vi "Main.vi"() -> ()   [LabVIEW 2024, in "FlexiFlowInterfaceCH2.lvlib"]
doc: "This template is based from the Queued Message Handler design pattern and the Queued Message Handler Project Template that ships with LabVIEW 2014.\n\nThe main difference is that the Queue is private to this module and communication between modules is done via Broadcast and Request events.\n\nRequest events are wrapped via public API methods and are handled in the Event handler loop in this VI.\nAny module can register for Broadcast events sent by this module.\n\nThe Event Handling Loop generates messages based on user interface actions.\n\nThe Message Handling Loop processes messages generated by the Event Handling Loop, or by other messages. The messages are string values, so new messages can be added easily to the Message Cases case structure in the Message Handling Loop. Each message cluster can also provide an optional value for Message Data, which is a variant that can be converted to whatever message-specific data is required.\n_____\nBased on Delacor QMH Project Template 3.1.0.34."
uses:
  FlexiFlowInterfaceCH2.lvlib
  <vilib>/Delacor/Delacor QMH/Libraries/Module Admin_class/Delacor_lib_QMH_Module Admin.lvclass
  <vilib>/MGI/Panel Manager/Panel/Panel/Panel.lvclass
  Module Data--cluster.ctl
  Modbus TCP Connection Settings--cluster.ctl
  Modbus Flexi-Flow State--cluster.ctl
  <vilib>/Plasmionique/MB Master/MB_Master_TCP/MB_Master_TCP.lvclass
  C:/Program Files/National Instruments/LabVIEW 2025/vi.lib/Plasmionique/MB Master/MB_Master/MB_Master.lvclass
  Device Type--enum.ctl
  Modbus Flexi-Flow Controls--cluster.ctl
  Modbus Flexi-Flow API/Control Mode--enum.ctl
  Modbus Flexi-Flow API/Control Function Values--enum.ctl
  Modbus Flexi-Flow Measure State--cluster.ctl
  <vilib>/Utility/miscctls.llb/LVPointTypeDef.ctl
  Initialise Modbus Connections Argument--cluster.ctl
  <vilib>/Delacor/Delacor QMH/Libraries/Message Queue_class/Delacor_lib_QMH_Message Queue.lvclass/Delacor_lib_QMH_Message Queue.ctl
  Stop Argument--cluster.ctl
  <vilib>/Delacor/Delacor QMH/Libraries/Module Admin_class/Delacor_lib_QMH_Module Admin.lvclass/Delacor_lib_QMH_Module Admin.ctl
  Read Fmeasure Argument--cluster.ctl
  FlexiFlowDevice--enum.ctl
  Set Modbus Configuration Argument--cluster.ctl
  Wink Devices Argument--cluster.ctl
  Read All FlexiFlow Device States Argument--cluster.ctl
  Wink Device Argument--cluster.ctl
  Set Control Function Argument--cluster.ctl
  Set Flow Setpoint Argument--cluster.ctl
  Set Backpressure Setpoint Argument--cluster.ctl
  Set Forward Pressure SP Argument--cluster.ctl
  Set Flow Capacity Unit Argument--cluster.ctl
  Modbus Flexi-Flow API/Capacity Units (Standard Volume Flow).ctl
  Set Setpoint Slope Argument--cluster.ctl
  Set Counter Settings Argument--cluster.ctl
  Counter Settings--cluster.ctl
  Modbus Flexi-Flow API/Counter Setpoint Mode--enum.ctl
  Modbus Flexi-Flow API/Counter Modes--enum.ctl
  Reset All Device Counters Argument--cluster.ctl
  Read Device User Tag Argument--cluster.ctl
  Set Device User Tag Argument--cluster.ctl
  Read Counter Unit Argument--cluster.ctl
  Set Control Mode Argument--cluster.ctl
  Get Device Configuration Argument--cluster.ctl
  Modbus Flexi-Flow API/PDU Address Float 32-bit Params--ring.ctl
  <vilib>/Delacor/Delacor QMH/Libraries/Message Queue_class/Delacor_lib_QMH_Enqueue Message (Single).vi
  <vilib>/Delacor/Delacor QMH/Libraries/Module Admin_class/Delacor_lib_QMH_Get External Launch.vi
  <vilib>/Utility/error.llb/Error Cluster From Error Code.vi
  <vilib>/ErrorRing/Error Ring.xnode
  <vilib>/Delacor/Delacor QMH/Libraries/Message Queue_class/Delacor_lib_QMH_Message Queue.lvclass
  <vilib>/MGI/Panel Manager/Panel/Panel Helper/Panel Helper.lvclass
  Modbus Flexi-Flow API/Bronkhorst Flexi-Flow ModbusTCP API.lvlib
panel:
  out "Counter Unit":string
  out "Read Capacity Unit":string
  out "Counters":sgl[](array[numeric])
  in  "Flexi-Flow Conn":T1[](array[typedef])=[{"Label"="hydrogen_inlet", "Slave ID (255)"=255, "IP Address"="192.168.100.10", "Port (502)"=502, "Timeout (10000)"=2000}, {"Label"="nitrogen_inlet", "Slave ID (255)"=255, "IP Address"="192.168.100.20", "Port (502)"=502, "Timeout (10000)"=2000}, {"Label"="cathode_outlet", "Slave ID (255)"=255, "IP Address"="192.168.100.30", "Port (502)"=502, "Timeout (10000)"=2000}, {"Label"="anode_outlet", "Slave ID (255)"=255, "IP Address"="192.168.100.40", "Port (502)"=502, "Timeout (10000)"=2000}]
  out "Data Cluster":T2 {"Flexi-Flow Devices"."Control State"."Control Mode" items=["Bus/RS232"=0, "FLOW-BUS slave"=2, "Valve close"=3, "Controller idle"=4, "Setpoint 100%"=7, "Valve fully open"=8, "Calibration mode"=9, "Setpoint 0%"=12, "RS232"=18, "Valve steering"=20, "Valve safe state"=22]}
  in  "Panel":refnum<class "Panel.lvclass">
  in  "Simulate MHL Error":bool
  in  "Simulate EHL Error":bool
  out "error out":errorcluster
  in  "Module Admin":refnum<class "Delacor_lib_QMH_Module Admin.lvclass">
  out "Status":string
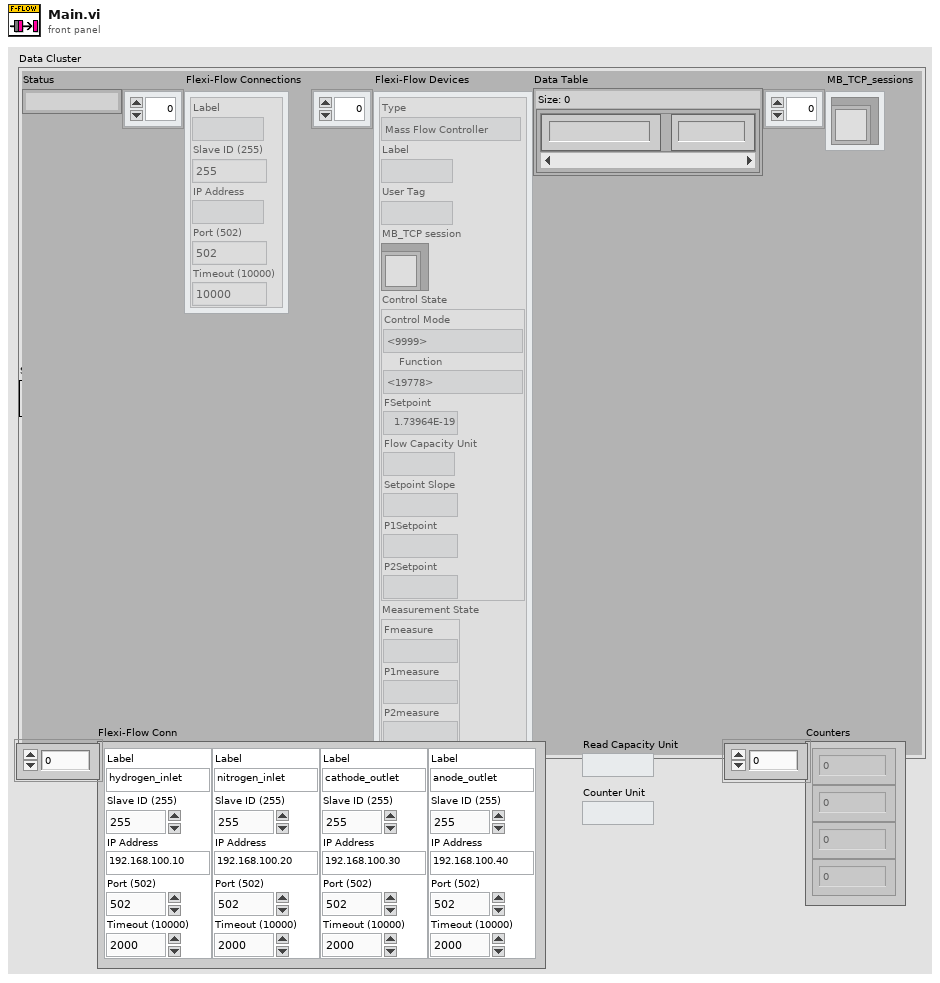
[diagram p1: front panel]
types:
  T1 = typedef "FlexiFlowInterfaceCH2.lvlib/Modbus TCP Connection Settings--cluster.ctl" = cluster{"Label":string, "Slave ID (255)":u8, "IP Address":string, "Port (502)":u16, "Timeout (10000)":i32}
  T2 = typedef "FlexiFlowInterfaceCH2.lvlib/Module Data--cluster.ctl" = cluster{"Status":string, "Flexi-Flow Connections":T1[], "Flexi-Flow Devices":T3[], "Data Table":map{string, dbl}, "MB_TCP_sessions":refnum<class "MB_Master_TCP.lvclass">[]}
  T3 = typedef "FlexiFlowInterfaceCH2.lvlib/Modbus Flexi-Flow State--cluster.ctl" = cluster{"Type":T4, "Label":string, "User Tag":string, "MB_TCP session":refnum<class "MB_Master_TCP.lvclass">, "Control State":T5, "Measurement State":T8}
  T4 = typedef "FlexiFlowInterfaceCH2.lvlib/Device Type--enum.ctl" = enum16{"Mass Flow Controller", "Mass Flow Meter"}
  T5 = typedef "FlexiFlowInterfaceCH2.lvlib/Modbus Flexi-Flow Controls--cluster.ctl" = cluster{"Control Mode":T6, "Function":T7, "FSetpoint":sgl, "Flow Capacity Unit":string, "Setpoint Slope":u16, "P1Setpoint":sgl, "P2Setpoint":sgl}
  T6 = typedef "Bronkhorst Flexi-Flow ModbusTCP API.lvlib/Control Mode--enum.ctl" = u16
  T7 = typedef "Bronkhorst Flexi-Flow ModbusTCP API.lvlib/Control Function Values--enum.ctl" = enum16{"Flow", "Upstream pressure", "Downstream pressure", "Flow with upstream pressure limit", "Flow with downstream pressure limit", "Upstream pressure with flow limit", "Downstream pressure with flow limit"}
  T8 = typedef "FlexiFlowInterfaceCH2.lvlib/Modbus Flexi-Flow Measure State--cluster.ctl" = cluster{"Fmeasure":dbl, "P1measure":sgl, "P2measure":sgl}
  T9 = typedef "LVPointTypeDef.ctl" = cluster{"Horizontal":i16, "Vertical":i16}
  T10 = typedef "FlexiFlowInterfaceCH2.lvlib/Request Events--cluster.ctl" = cluster{"Stop Module":refnum<user-event>, "Show Panel":refnum<user-event>, "Hide Panel":refnum<user-event>, "Get Module Execution Status":refnum<user-event>, "Show Diagram":refnum<user-event>, "Change Panel":refnum<user-event>, "Private":cluster{"Start Modbus Polling Helper Loop":refnum<user-event>, "Sleep Modbus Polling Helper Loop":refnum<user-event>, "Wake Connection Helper Loop":refnum<user-event>, "Sleep Connection Helper Loop":refnum<user-event>}, "Initialise Modbus Connections":refnum<user-event>, "Read Fmeasure":refnum<user-event>, "Set Modbus Configuration":refnum<user-event>, "Wink Devices":refnum<user-event>, "Read All FlexiFlow Device States":refnum<user-event>, "Wink Device":refnum<user-event>, "Set Control Function":refnum<user-event>, "Set Flow Setpoint":refnum<user-event>, "Set Backpressure Setpoint":refnum<user-event>, "Set Forward Pressure SP":refnum<user-event>, "Set Capacity Unit":refnum<user-event>, "Set Flow Capacity Unit":refnum<user-event>, "Set Setpoint Slope":refnum<user-event>, "Set Counter Settings":refnum<user-event>, "Reset All Device Counters":refnum<user-event>, "Read Device User Tag":refnum<user-event>, "Set Device User Tag":refnum<user-event>, "Read Counter Unit":refnum<user-event>, "Set Control Mode":refnum<user-event>, "Get Device Configuration":refnum<user-event>}
  T11 = typedef "Panel.lvlib/Panel Helper.lvclass/Panel Events.ctl" = cluster{"My Panel":refnum<user-event>, "Top Level Initialized":refnum<user-event>}
  T12 = typedef "FlexiFlowInterfaceCH2.lvlib/Initialise Modbus Connections Argument--cluster.ctl" = cluster{"Boolean":bool}
  T13 = typedef "FlexiFlowInterfaceCH2.lvlib/Stop Argument--cluster.ctl" = cluster{"Origin":string, "Exit via Stop Module Req?":bool, "Wait for Module to stop?":bool}
  T14 = typedef "FlexiFlowInterfaceCH2.lvlib/Read Fmeasure Argument--cluster.ctl" = cluster{"Device":T15}
  T15 = typedef "FlexiFlowInterfaceCH2.lvlib/FlexiFlowDevice--enum.ctl" = enum16{"Hydrogen Inlet", "Nitrogen Inlet", "Cathode Outlet", "Anode Outlet"}
  T16 = typedef "FlexiFlowInterfaceCH2.lvlib/Set Modbus Configuration Argument--cluster.ctl" = cluster{"Device":T15, "Modbus TCP Connection":T1}
  T17 = typedef "FlexiFlowInterfaceCH2.lvlib/Wink Devices Argument--cluster.ctl" = cluster{"Boolean":bool}
  T18 = typedef "FlexiFlowInterfaceCH2.lvlib/Read All FlexiFlow Device States Argument--cluster.ctl" = cluster{"Boolean":bool}
  T19 = typedef "FlexiFlowInterfaceCH2.lvlib/Wink Device Argument--cluster.ctl" = cluster{"Device":T15}
  T20 = typedef "FlexiFlowInterfaceCH2.lvlib/Set Control Function Argument--cluster.ctl" = cluster{"Device":T15, "Function":T7}
  T21 = typedef "FlexiFlowInterfaceCH2.lvlib/Set Flow Setpoint Argument--cluster.ctl" = cluster{"Device":T15, "Setpoint Value":dbl}
  T22 = typedef "FlexiFlowInterfaceCH2.lvlib/Set Backpressure Setpoint Argument--cluster.ctl" = cluster{"Device":T15, "Backpressure SP":dbl}
  T23 = typedef "FlexiFlowInterfaceCH2.lvlib/Set Forward Pressure SP Argument--cluster.ctl" = cluster{"Device":T15, "Pressure SP":dbl}
  T24 = typedef "FlexiFlowInterfaceCH2.lvlib/Set Flow Capacity Unit Argument--cluster.ctl" = cluster{"Device":T15, "Standard Volume Flow":T25}
  T25 = typedef "Bronkhorst Flexi-Flow ModbusTCP API.lvlib/Capacity Units (Standard Volume Flow).ctl" = u16
  T26 = typedef "FlexiFlowInterfaceCH2.lvlib/Set Setpoint Slope Argument--cluster.ctl" = cluster{"Setpoint Slope":u16, "Device":T15}
  T27 = typedef "FlexiFlowInterfaceCH2.lvlib/Set Counter Settings Argument--cluster.ctl" = cluster{"Device":T15, "Counter Settings":T28}
  T28 = typedef "FlexiFlowInterfaceCH2.lvlib/Counter Settings--cluster.ctl" = cluster{"Counter Setpoint Mode":T29, "Counter Limit":sgl, "Unit":string, "Counter Mode":T30, "Counter New Setpoint":u16}
  T29 = typedef "Bronkhorst Flexi-Flow ModbusTCP API.lvlib/Counter Setpoint Mode--enum.ctl" = enum16{"No setpoint change (default)", "Change setpoint to Counter new setpoint"}
  T30 = typedef "Bronkhorst Flexi-Flow ModbusTCP API.lvlib/Counter Modes--enum.ctl" = enum16{"Counter off (default)", "Counting up continuously", "Counting up until limit reached"}
  T31 = typedef "FlexiFlowInterfaceCH2.lvlib/Reset All Device Counters Argument--cluster.ctl" = cluster{"Boolean":bool}
  T32 = typedef "FlexiFlowInterfaceCH2.lvlib/Read Device User Tag Argument--cluster.ctl" = cluster{"Device":T15}
  T33 = typedef "FlexiFlowInterfaceCH2.lvlib/Set Device User Tag Argument--cluster.ctl" = cluster{"Device":T15, "User Tag":string}
  T34 = typedef "FlexiFlowInterfaceCH2.lvlib/Read Counter Unit Argument--cluster.ctl" = cluster{"Device":T15}
  T35 = typedef "FlexiFlowInterfaceCH2.lvlib/Set Control Mode Argument--cluster.ctl" = cluster{"Device":T15, "Control Mode":T6}
  T36 = typedef "FlexiFlowInterfaceCH2.lvlib/Get Device Configuration Argument--cluster.ctl" = cluster{"Device":T15}
  T37 = enum32{"invalid lock state", "Not Locked", "Locked (No Password)", "Password-protected"}
  T38 = enum16{"No reset", "Reset counter", "Reset alarm", "Reset counter (all)", "Reset and disable counter", "Reset firmware program (soft reset)", "Reset Alarm infor error bit", "Reset Alarm info warning bit"}
  T39 = typedef "Bronkhorst Flexi-Flow ModbusTCP API.lvlib/PDU Address Float 32-bit Params--ring.ctl" = u16
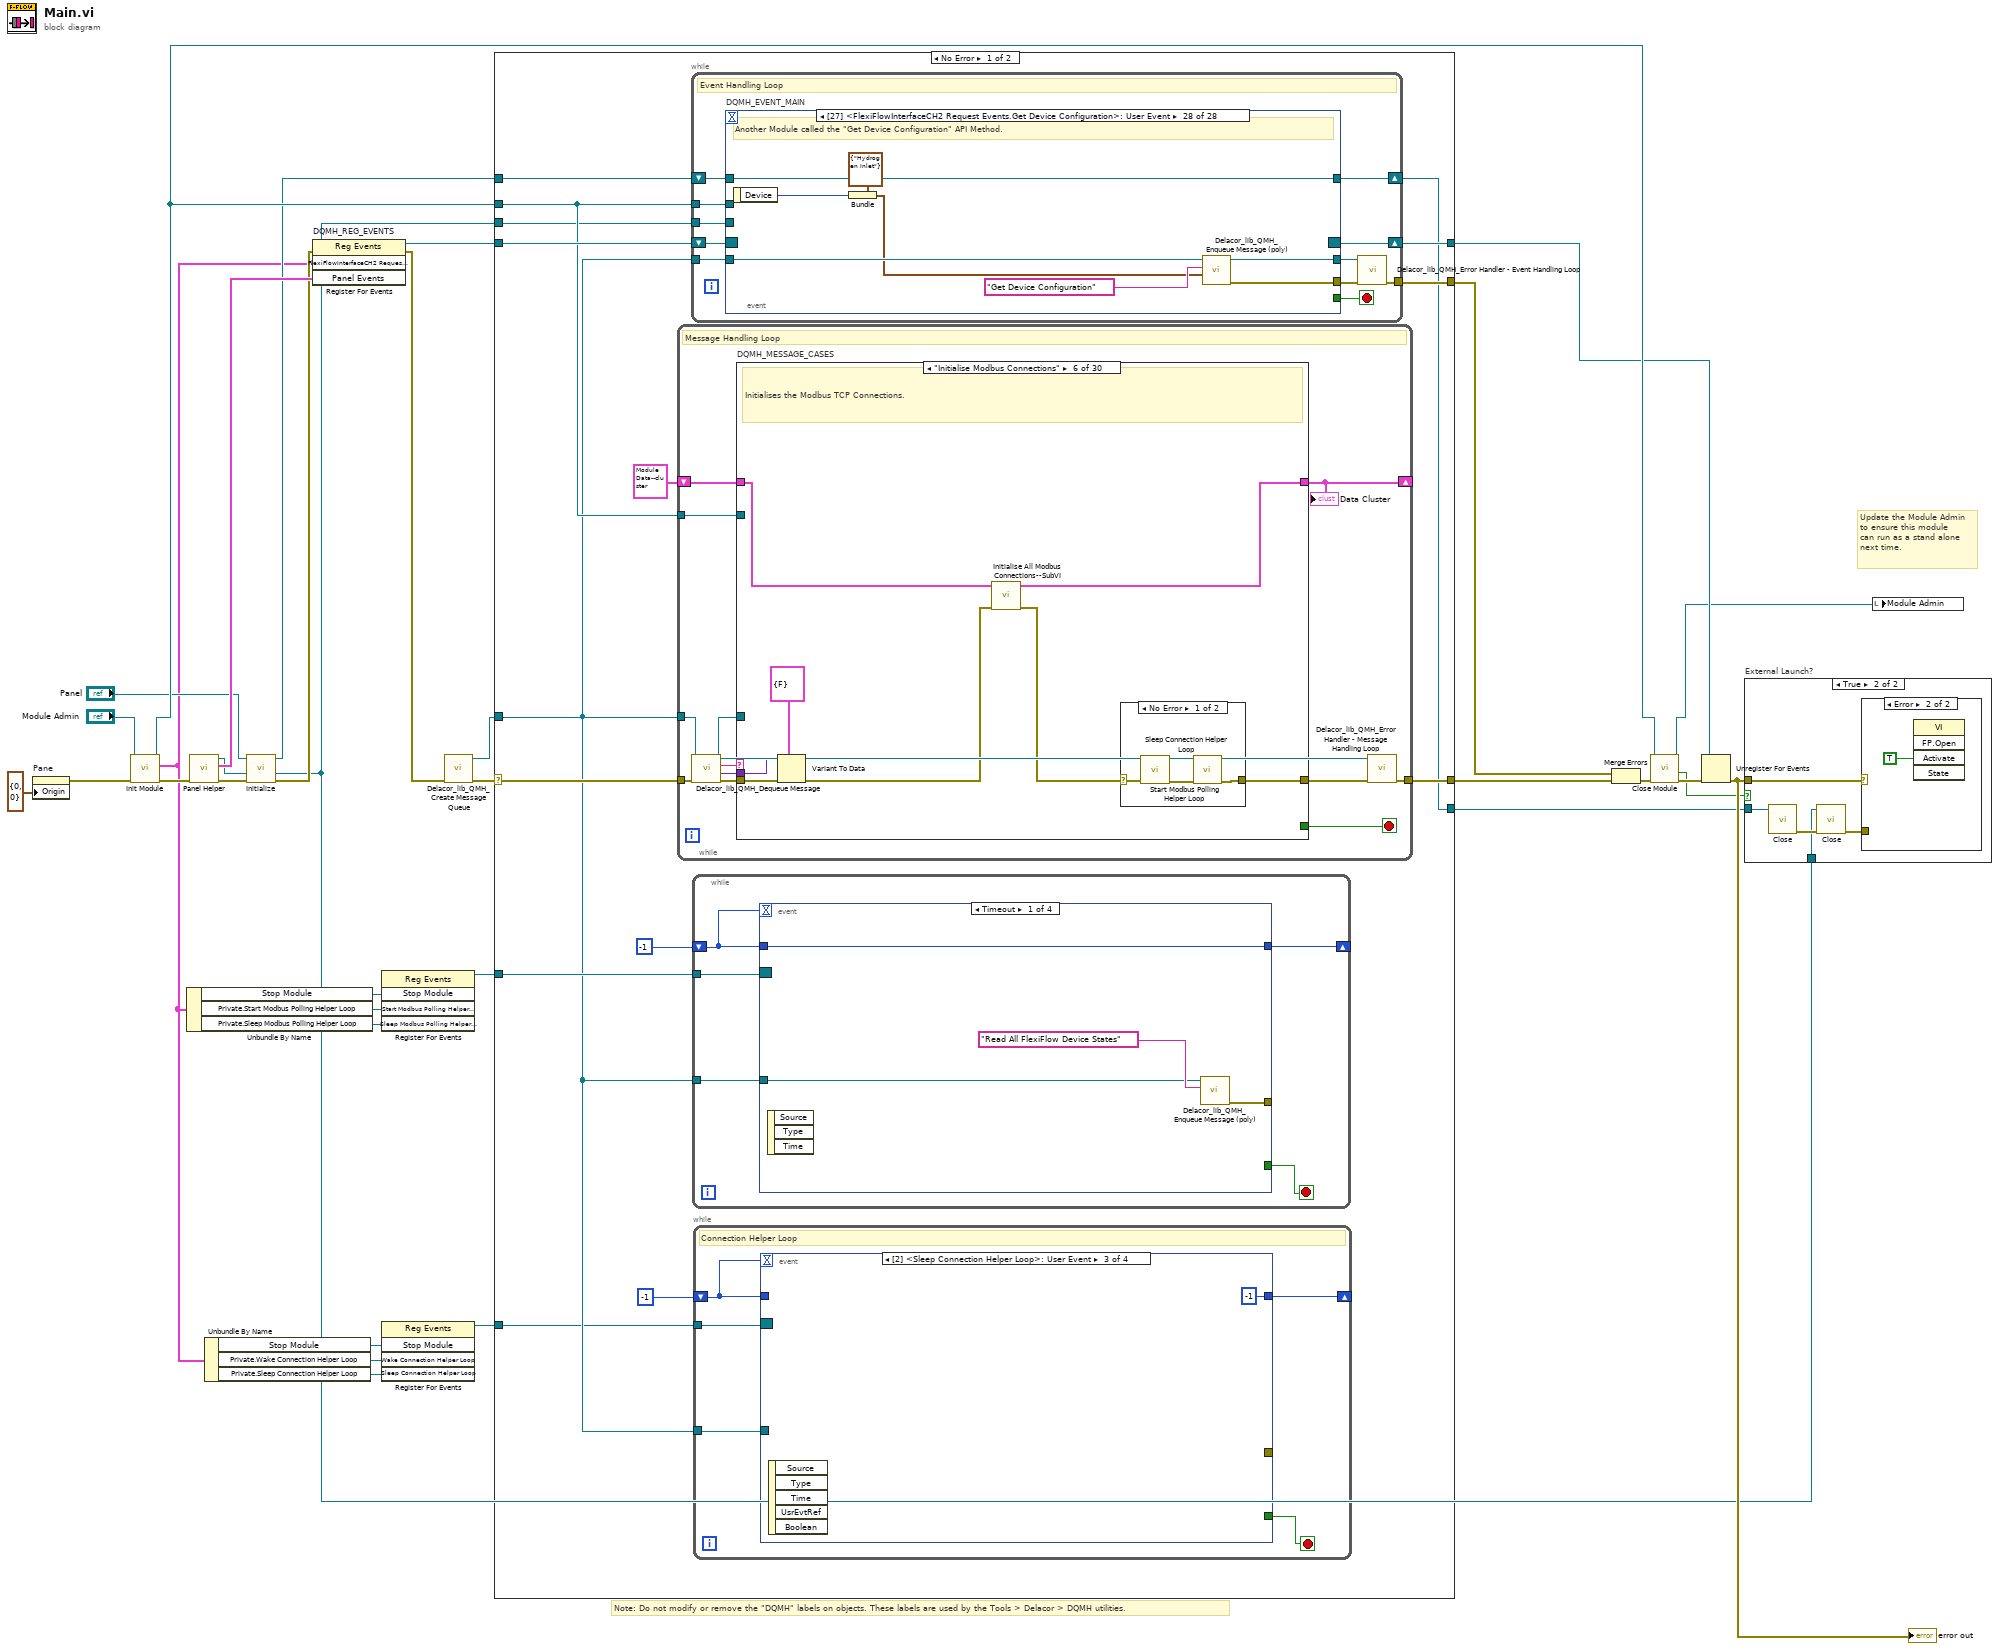
[diagram p0: block diagram]
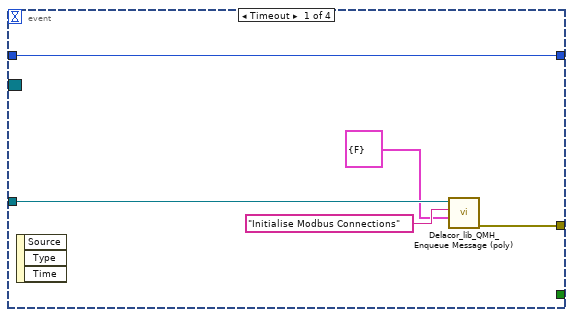
[diagram p4: hidden frame]
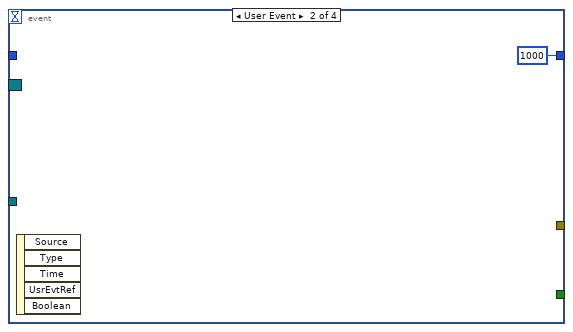
[diagram p5: hidden frame]
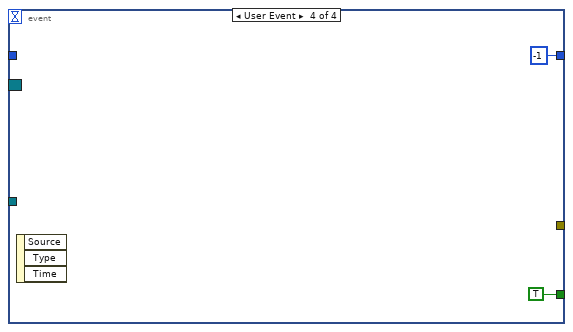
[diagram p6: hidden frame]
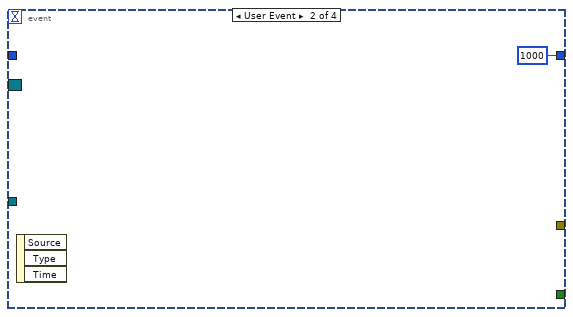
[diagram p7: hidden frame]
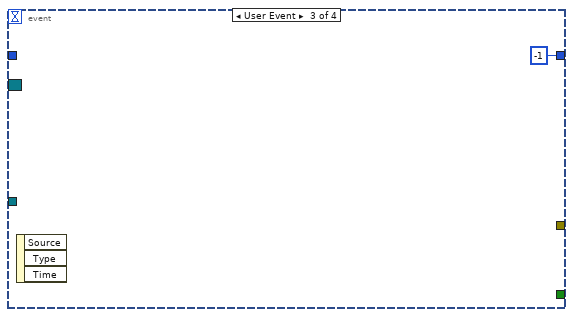
[diagram p8: hidden frame]
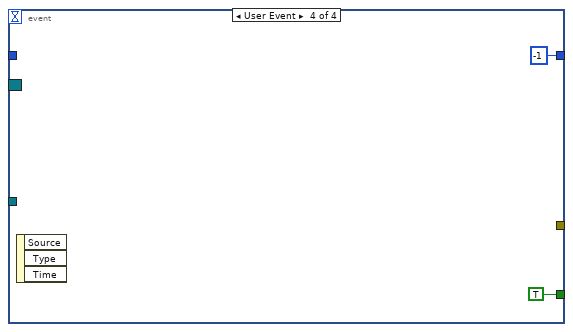
[diagram p9: hidden frame]
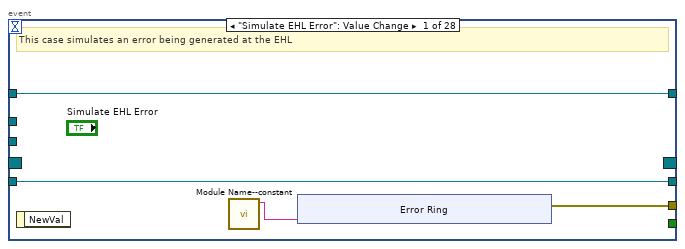
[diagram p10: hidden frame]
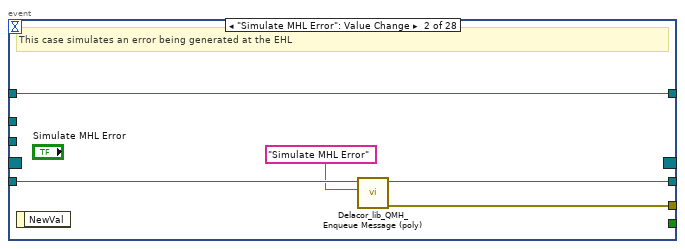
[diagram p11: hidden frame]
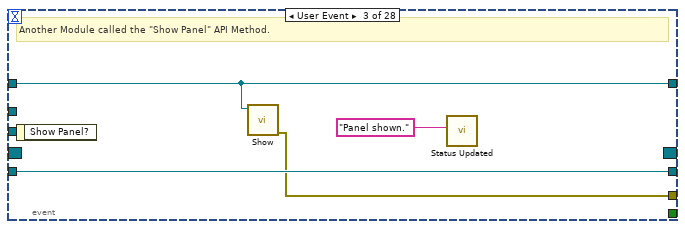
[diagram p12: hidden frame]
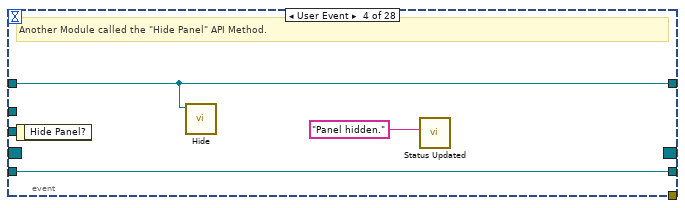
[diagram p13: hidden frame]
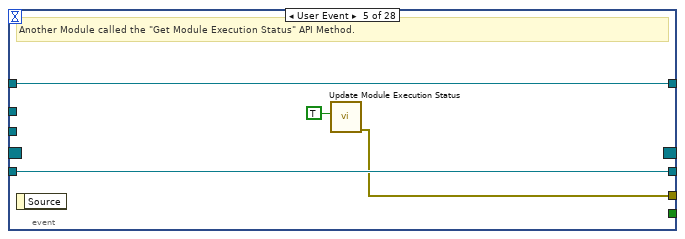
[diagram p14: hidden frame]
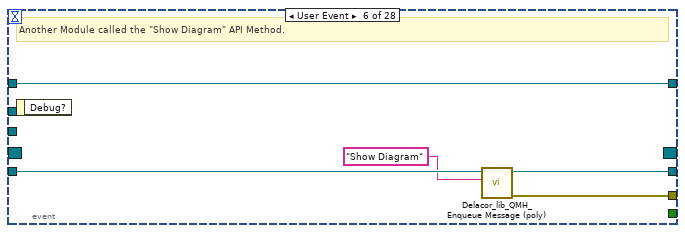
[diagram p15: hidden frame]
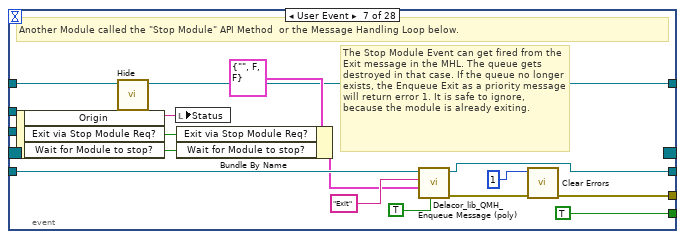
[diagram p16: hidden frame]
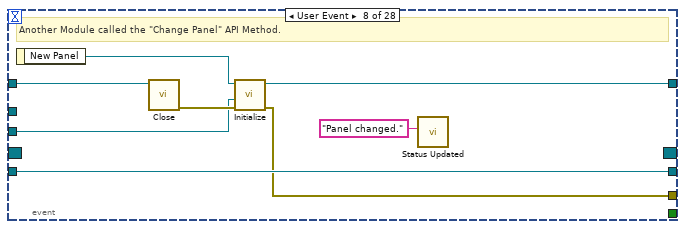
[diagram p17: hidden frame]
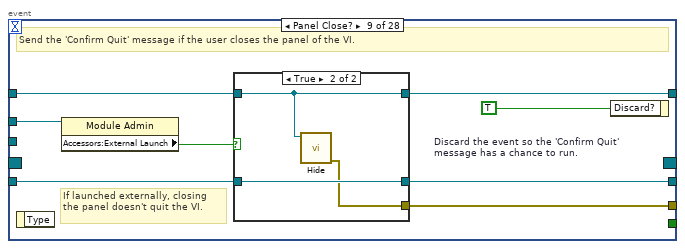
[diagram p18: hidden frame]
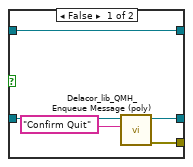
[diagram p19: hidden frame]
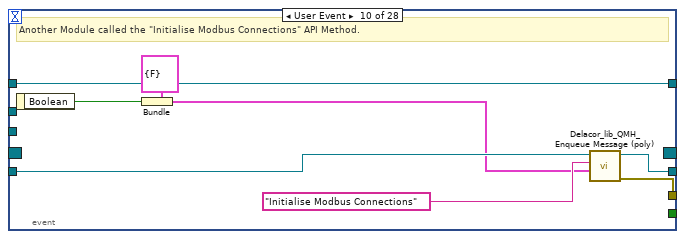
[diagram p20: hidden frame]
diagram:
  # "Note: Do not modify or remove the \"DQMH\" labels on objects. These labels are used by the Tools > Delacor > DQMH utilities."
  # "Update the Module Admin to ensure this module can run as a stand alone next time."
  n1 = property on="Pane" class="Pane"("Origin"=T9 {"Horizontal"=0, "Vertical"=0}) -> (error out=w10:errorcluster)  [unwired: 2 in, 1 out]
  n2 = call "Init Module.vi"("error in (no error)"=w10, "Singleton Module Admin in"="Module Admin") -> ("error out"=w20:errorcluster, "FlexiFlowInterfaceCH2 Request Events"=w5:T10, "Singleton Module Admin out"=w34:refnum<class "Delacor_lib_QMH_Module Admin.lvclass">)  [unwired: 7 in]
  n3 = Unbundle By Name(w5) -> ("Stop Module"=w8:refnum<user-event>, "Private.Start Modbus Polling Helper Loop"=w7:refnum<user-event>, "Private.Sleep Modbus Polling Helper Loop"=w6:refnum<user-event>)
  n4 = call <vilib>:"Panel Helper.vi"("Error In"=w20) -> ("Error Out"=w17:errorcluster, "Panel Events"=w19:T11, "Panel Helper out"=w16:refnum<class "Panel Helper.lvclass">)  [unwired: 8 in]
  n5 = Unbundle By Name(w5) -> ("Stop Module"=w4:refnum<user-event>, "Private.Wake Connection Helper Loop"=w3:refnum<user-event>, "Private.Sleep Connection Helper Loop"=w1:refnum<user-event>)
  n6 = call <vilib>:"Initialize.vi"("error in (no error)"=w17, "My Helper in"=w16, "Panel In"="Panel") -> ("error out"=w14:errorcluster, "My Helper out"=w13:refnum<class "Panel Helper.lvclass">, "Panel Out"=w12:refnum<class "Panel.lvclass">)  [unwired: 6 in]
  n7 = register-events "DQMH_REG_EVENTS"(error in=w14, w5, w19) -> (reference out=w31:refnum<event-registration>, error out=w18:errorcluster)  [unwired: 1 in]
  n8 = register-events(w8, w7, w6) -> (reference out=w9:refnum<event-registration>)  [unwired: 2 in, 1 out]
  n9 = register-events(w4, w3, w1) -> (reference out=w2:refnum<event-registration>)  [unwired: 2 in, 1 out]
  n10 = call <vilib>:"Delacor_lib_QMH_Create Message Queue.vi"("error in"=w18) -> ("error out"=w22:errorcluster, "Message Queue"=w30:refnum<class "Delacor_lib_QMH_Message Queue.lvclass">)  [unwired: 9 in]
  n11 = case shown="No Error" w22 {
    selector: w22 -> [w44 w707]
    tunnel: [w49 w707] -> w33
    tunnel: [w48 w712] -> w32
    tunnel: w31 -> [w46 w712]
    tunnel: w30 -> [w36 _]
    tunnel: [w45 _] -> w26
    tunnel: w34 -> [w43 w708]
    tunnel: w12 -> [w41 w704]
    tunnel: w13 -> [w42 _]
    tunnel: [w40 w704] -> w21
    tunnel: w9 -> [w38 _]
    tunnel: w2 -> [w35 _]
    frame No Error {
      n12 = while {
        tunnel: w36 -> [w324]
        shift-right: [w320] -> _
        shift-left: T2 {"Status"="", "Flexi-Flow Connections"=[], "Flexi-Flow Devices"=[], "Data Table"={}, "MB_TCP_sessions"=[]} ("Data Cluster") -> [w330]
        tunnel: w44 -> [w328]
        tunnel: [w322] -> w49
        tunnel: w43 -> [w321]
        stop <- w329 stop-if-true
        # "Message Handling Loop"
        n13 = call-dynamic "Delacor_lib_QMH_Dequeue Message.vi"("error in"=w328, "Message Queue in"=w324) -> ("error out"=w327:errorcluster, "Message Data"=w325:variant, "Message"=w326:string, "Message Queue out"=w323:refnum<class "Delacor_lib_QMH_Message Queue.lvclass">)  [unwired: 6 in]
        n14 = case "DQMH_MESSAGE_CASES" shown="\"Initialise Modbus Connections\"" w326 {
          selector: w326 -> [_ _ _ _ _ _ _ _ _ _ _ _ _ _ _ _ _ _ _ _ _ _ _ _ _ _ _ _ _ w694]
          tunnel: w323 -> [_ _ _ _ _ _ _ _ _ _ _ _ _ _ _ _ _ _ _ _ _ _ _ _ _ _ w654 w669 w687 _]
          tunnel: w327 -> [w341 w351 w355 w372 w378 w386 w399 w412 w428 w441 w457 w476 w495 w506 w516 w524 w543 w552 w574 w588 w602 w617 w631 w634 w637 w642 w659 w672 w689 _]
          tunnel: [w342 w352 w354 w371 w377 w380 w396 w407 w423 w437 w450 w467 w485 w502 w510 w520 w536 w544 w566 w578 w590 w604 w618 w633 w636 w641 w651 w671 w684 w695] -> w331
          tunnel: w330 -> [w338 w345 w353 w370 w373 w382 w394 w405 w420 w436 w453 w469 w484 w498 w512 w523 w539 w549 w568 w582 w596 w609 w625 w632 w635 w638 w650 w666 w675 w692]
          tunnel: [_ _ _ _ _ _ _ _ _ _ _ _ _ _ _ _ _ _ _ _ _ _ _ _ _ _ _ _ w686 _] -> w329
          tunnel: w325 -> [_ w350 _ _ w376 w385 w398 w411 w427 w440 w456 w475 w494 w505 w515 w526 w542 w551 w573 w587 w601 w616 w630 _ _ _ w658 _ w683 _]
          tunnel: w321 -> [w339 _ _ _ _ _ _ _ _ _ _ _ _ _ _ _ _ _ _ _ _ _ _ _ _ _ w653 _ w678 _]
          tunnel: [w336 w345 w353 w370 w373 w381 w393 w404 w418 w430 w449 w463 w483 w500 w508 w522 w538 w548 w563 w581 w595 w608 w624 w632 w635 w638 w650 w666 w675 w692] -> w320
          frame "Initialize" {
            w337 = "Initial Message" ("Initial Message")
            # "Initialize - Any operation that needs to be done before the module can receive messages. Synchronize Caller Events.vi will inform Start Module.vi that the module has launched and is ready to receive messages. Module Did Init.vi will broadcast that the module initialized."
            n15 = Array Size(array="Flexi-Flow Conn") -> (size(s)=w333:i32)
            n16 = local write "Status"(w337) -> ()
            n17 = Initialize Array(T3 {"Type"=enum."Mass Flow Controller", "Label"="", "User Tag"="", "MB_TCP session"=refnum, "Control State"={"Control Mode"=0, "Function"=enum."Flow", "FSetpoint"=0.0, "Flow Capacity Unit"="", "Setpoint Slope"=0, "P1Setpoint"=0.0, "P2Setpoint"=0.0}, "Measurement State"={"Fmeasure"=0.0, "P1measure"=0.0, "P2measure"=0.0}} ("Flexi-Flow"), w333) -> (w332:T3[])
            n18 = call "Synchronize Caller Events.vi"("error in (no error)"=w341, "Singleton Module Admin in"=w339) -> ("error out"=w340:errorcluster)  [unwired: 8 in, 1 out]
            n19 = Bundle By Name(cluster=w338, "Status"=w337, "Flexi-Flow Connections"="Flexi-Flow Conn", "Flexi-Flow Devices"=w332) -> (w336:T2)
            n20 = call "Module Name--constant.vi"() -> ("Module Name"=w343:string)  [unwired: 11 in]
            n21 = call "Module Did Init.vi"("error in (no error)"=w340, "Initialized?"=TRUE, "Origin"=w343) -> ("error out"=w342:errorcluster)  [unwired: 8 in]
          }
          frame "Update Display" {
            # "Broadcast updated status to any VI registered to listen to this module's broadcast events."
            # "Convert the message data to a string to display in the Status indicator."
            # "#CodeRecommended - If you wish to decouple the Message Handling Loop from your user interface, consider creating User Events (like the \"Stop\" event in this VI) to message the Event Handling Loop whenever the user interface needs updating."
            # "Update Display - Update user interface here."
            n22 = Variant To Data(error in=w351, type="" ("Empty String Constant"), Variant=w350) -> (data=w348:string, error out=w347:errorcluster)
            "Status" <- w348
            n23 = call "Status Updated.vi"("error in (no error)"=w347, "Status"=w348) -> ("error out"=w346:errorcluster)  [unwired: 9 in]
            n24 = Merge Errors(w346) -> (w352:errorcluster)
          }
          frame "Show Diagram" {
            # "Show Diagram - Show the block diagram of this VI. Used as a debugging tool. There is a button in the module tester that fires the Show Diagram request, which runs this message. Note that the diagram will not be displayed if it is password-protected and the password is not in the cache."
            n25 = disable-structure shown="RUN_TIME_ENGINE==False" {
              disable-tunnel: [w363 w369] -> w354
              disable-tunnel: w355 -> [w362 w369]
              frame condition #0 (active) {
                # "functionality not available in exe"
                n26 = invoke class="VI" method="Lock State.Get"(error in=w362) -> (error out=w361:errorcluster, "Get Lock State"=w360:T37, "pwd in cache"=w357:bool)  [unwired: 3 in, 1 out]
                n27 = Equal?(x=T37."Password-protected", y=w360) -> (x = y?=w358:bool)
                n28 = Compound Arithmetic op=AND(w358, invert w357) -> (w356:bool)
                n29 = case shown="False" w356 {
                  tunnel: [w366 w368] -> w363
                  tunnel: w361 -> [w364 w368]
                  frame False {
                    n30 = property class="VI"(error in=w364, "BDWin.Open"=TRUE ("Block Diagram Window:Open")) -> (error out=w366:errorcluster)  [unwired: 1 in, 1 out]
                    n31 = call "Status Updated.vi"("Status"="Block Diagram shown." ("format string")) -> ()  [unwired: 10 in, 1 out]
                  }
                  frame True {
                    # "Password-protected VI, and the password is not in the cache. Do not show the diagram."
                  }
                }
              }
              frame condition #1 {
              }
            }
          }
          frame "--- Module Specific ---" {
            # "Separator -- The following cases handle messages specific to this Module."
            n32 = Merge Errors(w372) -> (w371:errorcluster)
          }
          frame "Set Modbus Configuration" {
            # "Sets the modbus configuration."
            n33 = Variant To Data(error in=w378, type=T16 {"Device"=enum."Hydrogen Inlet", "Modbus TCP Connection"={"Label"="", "Slave ID (255)"=255, "IP Address"="", "Port (502)"=502, "Timeout (10000)"=10000}} ("Set Modbus Configuration Argument"), Variant=w376) -> (data=w374:T16, error out=w377:errorcluster)
            n34 = Unbundle By Name(w374) -> ()  [unwired: 2 out]
          }
          frame "Initialise Modbus Connections" {
            # "Initialises the Modbus TCP Connections."
            n35 = Variant To Data(error in=w386, type=T12 {"Boolean"=FALSE} ("Initialise Modbus Connections Argument"), Variant=w385) -> (error out=w383:errorcluster)  [unwired: 1 out]
            n36 = call "Initialise All Modbus Connections--SubVI.vi"("error in (no error)"=w383, "Data Cluster in"=w382) -> ("error out"=w379:errorcluster, "Data Cluster out"=w381:T2)  [unwired: 8 in]
            n37 = case shown="No Error" w379 {
              selector: w379 -> [w388 w392]
              tunnel: [w389 w390] -> w380
              frame No Error {
                n38 = call "Sleep Connection Helper Loop.vi"("error in"=w388) -> ("error out"=w387:errorcluster)  [unwired: 10 in]
                n39 = call "Start Modbus Polling Helper Loop.vi"("error in"=w387) -> ("error out"=w389:errorcluster)  [unwired: 10 in]
              }
              frame Error {
                n40 = call "Sleep Modbus Polling Helper Loop.vi"("error in"=w392) -> ("error out"=w391:errorcluster)  [unwired: 10 in]
                n41 = call "Wake Connection Helper Loop.vi"("error in"=w391) -> ("error out"=w390:errorcluster)  [unwired: 10 in]
              }
            }
          }
          frame "Wink Devices" {
            # "Wink the flexi-flow devices."
            n42 = Variant To Data(error in=w399, type=T17 {"Boolean"=FALSE} ("Wink Devices Argument"), Variant=w398) -> (error out=w395:errorcluster)  [unwired: 1 out]
            n43 = call "Wink Devices--SubVI.vi"("error in (no error)"=w395, "Data Cluster in"=w394) -> ("error out"=w396:errorcluster, "Data Cluster out"=w393:T2)  [unwired: 8 in]
          }
          frame "Wink Device" {
            # "Winks the specified FlexiFlow device."
            n44 = Variant To Data(error in=w412, type=T19 {"Device"=enum."Hydrogen Inlet"} ("Wink Device Argument"), Variant=w411) -> (data=w409:T19, error out=w408:errorcluster)
            n45 = Unbundle By Name(w409) -> ("Device"=w400:T15)
            n46 = call "Get Device Modbus TCP Session.vi"("Device"=w400, "Data Cluster In"=w405) -> ("Device State"=w401:T3, "MB_TCP session"=w402:refnum<class "MB_Master_TCP.lvclass">, "Data Cluster Out"=w406:T2)  [unwired: 7 in]
            n47 = call "Wink.vi"("error in"=w408, "MB_TCP session in"=w402) -> ("error out"=w407:errorcluster, "MB session out"=w403:refnum<class "MB_Master_TCP.lvclass">)  [unwired: 8 in]
            n48 = call "Update Device.vi"("Device"=w400, "Device State"=w401, "MB_TCP session"=w403, "Data Cluster"=w406) -> ("Data Cluster Out"=w404:T2)  [unwired: 7 in]
          }
          frame "Set Control Function" {
            # "Sets the control function."
            n49 = Variant To Data(error in=w428, type=T20 {"Device"=enum."Hydrogen Inlet", "Function"=enum."Flow"} ("Set Control Function Argument"), Variant=w427) -> (data=w425:T20, error out=w424:errorcluster)
            n50 = Unbundle By Name(w425) -> ("Device"=w414:T15, "Function"=w422:T7)
            n51 = call "Get Device Modbus TCP Session.vi"("Device"=w414, "Data Cluster In"=w420) -> ("Device State"=w416:T3, "MB_TCP session"=w415:refnum<class "MB_Master_TCP.lvclass">, "Data Cluster Out"=w421:T2)  [unwired: 7 in]
            n52 = call "Write Control Function.vi"("error in"=w424, "Function"=w422, "MB_TCP session in"=w415) -> ("error out"=w423:errorcluster, "Value"=w419:u16, "MB session out"=w413:refnum<class "MB_Master_TCP.lvclass">)  [unwired: 6 in]
            n53 = Bundle By Name(cluster=w416, "Control State.Function"=w419) -> (w417:T3)
            n54 = call "Update Device.vi"("Device"=w414, "Device State"=w417, "MB_TCP session"=w413, "Data Cluster"=w421) -> ("Data Cluster Out"=w418:T2)  [unwired: 7 in]
          }
          frame "Set Counter Settings" {
            # "Set the counter settings."
            n55 = Variant To Data(error in=w441, type=T27 {"Device"=enum."Hydrogen Inlet", "Counter Settings"={"Counter Setpoint Mode"=enum."No setpoint change (default)", "Counter Limit"=0.0, "Unit"="ls", "Counter Mode"=enum."Counter off (default)", "Counter New Setpoint"=0}} ("Set Counter Settings Argument"), Variant=w440) -> (data=w432:T27, error out=w438:errorcluster)
            n56 = Unbundle By Name(w432) -> ("Device"=w431:T15)
            n57 = call "Get Device Modbus TCP Session.vi"("Device"=w431, "Data Cluster In"=w436) -> ("Device State"=w434:T3, "MB_TCP session"=w429:refnum<class "MB_Master_TCP.lvclass">, "Data Cluster Out"=w435:T2)  [unwired: 7 in]
            n58 = call "Set Counter Settings--SubVI.vi"("error in (no error)"=w438, "Set Counter Settings Argument"=w432, "MB_Master_TCP in"=w429) -> ("error out"=w437:errorcluster, "MB_Master_TCP out"=w433:refnum<class "MB_Master_TCP.lvclass">)  [unwired: 7 in]
            n59 = call "Update Device.vi"("Device"=w431, "Device State"=w434, "MB_TCP session"=w433, "Data Cluster"=w435) -> ("Data Cluster Out"=w430:T2)  [unwired: 7 in]
          }
          frame "Set Flow Setpoint" {
            # "Sets the control value setpoint."
            n60 = Variant To Data(error in=w457, type=T21 {"Device"=enum."Hydrogen Inlet", "Setpoint Value"=0.0} ("Set Control Value SP Argument"), Variant=w456) -> (data=w454:T21, error out=w451:errorcluster)
            n61 = Unbundle By Name(w454) -> ("Device"=w444:T15, "Setpoint Value"=w452:dbl)
            n62 = call "Get Device Modbus TCP Session.vi"("Device"=w444, "Data Cluster In"=w453) -> ("Device State"=w446:T3, "MB_TCP session"=w445:refnum<class "MB_Master_TCP.lvclass">, "Data Cluster Out"=w448:T2)  [unwired: 7 in]
            n63 = call "Write Fsetpoint (Channel F).vi"("error in"=w451, "Value"=w452, "MB_TCP session in"=w445) -> ("error out"=w450:errorcluster, "Value"=w447:sgl, "MB session out"=w442:refnum<class "MB_Master_TCP.lvclass">)  [unwired: 6 in]
            n64 = Bundle By Name(cluster=w446, "Control State.FSetpoint"=w447) -> (w443:T3)
            n65 = call "Update Device.vi"("Device"=w444, "Device State"=w443, "MB_TCP session"=w442, "Data Cluster"=w448) -> ("Data Cluster Out"=w449:T2)  [unwired: 7 in]
          }
          frame "Set Backpressure Setpoint" {
            w465 = T39 41496 items=["FSetpoint (Channel F)"=41240, "Fmeasure (Channel F)"=41216, "FSetpoint (Channel P1)"=41496, "Fmeasure (Channel P1)"=41472, "FSetpoint (Channel P2)"=41752, "Fmeasure (Channel P2)"=41728, "Capacity 0%"=41392, "Counter limit (Float)"=59416, "Inlet Pressure"=61801, "Outlet Pressure"=61809, "PID-Kp"=62120, "PID-Ti"=62128, "PID-Td"=62136, "Dynamic display factor"=62728, "Static display factor"=62736, "Exponential smoothing"=62752] ("PDU Address 32-bit Float")
            # "Sets the backpressure setpoint (P1 - upstream) of the pressure regulator."
            n66 = Variant To Data(error in=w476, type=T22 {"Device"=enum."Cathode Outlet", "Backpressure SP"=0.0} ("Set Backpressure Setpoint Argument"), Variant=w475) -> (data=w473:T22, error out=w472:errorcluster)
            n67 = Unbundle By Name(w473) -> ("Device"=w462:T15, "Backpressure SP"=w471:dbl)
            n68 = call "Get Device Modbus TCP Session.vi"("Device"=w462, "Data Cluster In"=w469) -> ("Device State"=w461:T3, "MB_TCP session"=w460:refnum<class "MB_Master_TCP.lvclass">, "Data Cluster Out"=w470:T2)  [unwired: 7 in]
            n69 = call "Write Float Register.vi"("PDU Address 32-bit Float"=w465, "error in"=w472, "Value"=w471, "MB_TCP session in"=w460) -> ("error out"=w468:errorcluster, "MB session out"=w466:refnum<class "MB_Master_TCP.lvclass">)  [unwired: 6 in]
            n70 = call "Read Float Register.vi"("PDU Address 32-bit Float"=w465, "error in"=w468, "MB_TCP session in"=w466) -> ("error out"=w467:errorcluster, "Value"=w464:sgl, "MB session out"=w459:refnum<class "MB_Master_TCP.lvclass">)  [unwired: 6 in]
            n71 = Bundle By Name(cluster=w461, "Control State.P1Setpoint"=w464) -> (w458:T3)
            n72 = call "Update Device.vi"("Device"=w462, "Device State"=w458, "MB_TCP session"=w459, "Data Cluster"=w470) -> ("Data Cluster Out"=w463:T2)  [unwired: 7 in]
          }
          frame "Set Forward Pressure SP" {
            w482 = T39 41752 items=["FSetpoint (Channel F)"=41240, "Fmeasure (Channel F)"=41216, "FSetpoint (Channel P1)"=41496, "Fmeasure (Channel P1)"=41472, "FSetpoint (Channel P2)"=41752, "Fmeasure (Channel P2)"=41728, "Capacity 0%"=41392, "Counter limit (Float)"=59416, "Inlet Pressure"=61801, "Outlet Pressure"=61809, "PID-Kp"=62120, "PID-Ti"=62128, "PID-Td"=62136, "Dynamic display factor"=62728, "Static display factor"=62736, "Exponential smoothing"=62752] ("PDU Address 32-bit Float")
            # "Sets the forward pressure setpoint."
            n73 = Variant To Data(error in=w495, type=T23 {"Device"=enum."Hydrogen Inlet", "Pressure SP"=0.0} ("Set Forward Pressure SP Argument"), Variant=w494) -> (data=w492:T23, error out=w486:errorcluster)
            n74 = Unbundle By Name(w492) -> ("Device"=w480:T15, "Pressure SP"=w487:dbl)
            n75 = call "Get Device Modbus TCP Session.vi"("Device"=w480, "Data Cluster In"=w484) -> ("Device State"=w479:T3, "MB_TCP session"=w481:refnum<class "MB_Master_TCP.lvclass">, "Data Cluster Out"=w491:T2)  [unwired: 7 in]
            n76 = call "Write Float Register.vi"("PDU Address 32-bit Float"=w482, "error in"=w486, "Value"=w487, "MB_TCP session in"=w481) -> ("error out"=w490:errorcluster, "MB session out"=w489:refnum<class "MB_Master_TCP.lvclass">)  [unwired: 6 in]
            n77 = call "Read Float Register.vi"("PDU Address 32-bit Float"=w482, "error in"=w490, "MB_TCP session in"=w489) -> ("error out"=w485:errorcluster, "Value"=w488:sgl, "MB session out"=w477:refnum<class "MB_Master_TCP.lvclass">)  [unwired: 6 in]
            n78 = Bundle By Name(cluster=w479, "Control State.P2Setpoint"=w488) -> (w478:T3)
            n79 = call "Update Device.vi"("Device"=w480, "Device State"=w478, "MB_TCP session"=w477, "Data Cluster"=w491) -> ("Data Cluster Out"=w483:T2)  [unwired: 7 in]
          }
          frame "Set Flow Capacity Unit" {
            # "Sets the flow capacity unit."
            n80 = Variant To Data(error in=w506, type=T24 {"Device"=enum."Hydrogen Inlet", "Standard Volume Flow"=0} ("Set Flow Capacity Unit Argument"), Variant=w505) -> (data=w503:T24, error out=w501:errorcluster)
            n81 = Unbundle By Name(w503) -> ("Device"=w497:T15, "Standard Volume Flow"=w496:T25)
            n82 = call "Set Flow Capacity Unit--SubVI.vi"("error in (no error)"=w501, "Standard Volume Flow"=w496, "Device"=w497, "Data Cluster"=w498) -> ("error out"=w502:errorcluster, "Value"=→"Read Capacity Unit":string, "Data Cluster Out"=w500:T2)  [unwired: 5 in]
          }
          frame "Set Setpoint Slope" {
            # "Sets the setpoint slope in seconds. 0 to 3000 seconds. 0 is default. 10 corresponds to a change from 0 to 100% over 10 seconds."
            n83 = Variant To Data(error in=w516, type=T26 {"Setpoint Slope"=0, "Device"=enum."Hydrogen Inlet"} ("Set Setpoint Slope Argument"), Variant=w515) -> (data=w513:T26, error out=w511:errorcluster)
            n84 = Unbundle By Name(w513) -> ("Device"=w509:T15, "Setpoint Slope"=w507:u16)
            n85 = call "Set Setpoint Slope--SubVI.vi"("error in (no error)"=w511, "Setpoint Slope"=w507, "Device"=w509, "Data Cluster"=w512) -> ("error out"=w510:errorcluster, "Data Cluster Out"=w508:T2)  [unwired: 6 in]
          }
          frame "Read All FlexiFlow Device States" {
            # "Reads all Flex-Flow device states."
            n86 = Variant To Data(error in=w524, type=T18 {"Boolean"=FALSE} ("Read All FlexiFlow Device States Argument"), Variant=w526) -> ()  [unwired: 2 out]
            n87 = call "Read All Devices States.vi"("error in (no error)"=w524, "Data Cluster"=w523) -> ("error out"=w517:errorcluster, "Array"=→"Counters":sgl[], "Data Table"=w519:map{string, dbl}, "Array Out"=w521:T3[])  [unwired: 6 in]
            n88 = case shown="Error .." w517 {
              selector: w517 -> [w527 w534]
              tunnel: w521 -> [w531 _]
              tunnel: [w529 w532] -> w520
              tunnel: w519 -> [w528 _]
              frame No Error {
                n89 = call "Broadcast Device States.vi"("error in"=w527, "Flexi-Flow Devices"=w531) -> ("error out"=w530:errorcluster)  [unwired: 9 in]
                n90 = call "Broadcast State (Data Map).vi"("error in"=w530, "Data Table"=w528) -> ("error out"=w529:errorcluster)  [unwired: 9 in]
              }
              frame Error {
                n91 = call "Wake Connection Helper Loop.vi"("error in"=w534) -> ("error out"=w533:errorcluster)  [unwired: 10 in]
                n92 = call "Sleep Modbus Polling Helper Loop.vi"("error in"=w533) -> ("error out"=w532:errorcluster)  [unwired: 10 in]
              }
            }
            n93 = Bundle By Name(cluster=w523, "Flexi-Flow Devices"=w521, "Data Table"=w519) -> (w522:T2)
          }
          frame "Read Measure" {
            n94 = Variant To Data(error in=w543, type=T14 {"Device"=enum."Hydrogen Inlet"} ("Read Device State Argument"), Variant=w542) -> (data=w540:T14, error out=w537:errorcluster)
            n95 = Unbundle By Name(w540) -> ("Device"=w535:T15)
            n96 = call "Read Measure--SubVI.vi"("error in (no error)"=w537, "Device"=w535, "Data Cluster"=w539) -> ("error out"=w536:errorcluster, "Data Cluster Out"=w538:T2)  [unwired: 7 in]
          }
          frame "Reset All Device Counters" {
            # "Resets all device counters."
            n97 = Variant To Data(error in=w552, type=T31 {"Boolean"=FALSE} ("Reset All Device Counters Argument"), Variant=w551) -> (error out=w545:errorcluster)  [unwired: 1 out]
            n98 = Unbundle By Name(w549) -> ("Flexi-Flow Devices"=w547:T3[])
            n99 = for {
              tunnel: w547 -> [w558] mode=indexing
              tunnel: [w556] -> w546 mode=indexing
              tunnel: w545 -> [w554]
              tunnel: [w553] -> w544
              n100 = Unbundle By Name(w558) -> ("MB_TCP session"=w559:refnum<class "MB_Master_TCP.lvclass">)
              n101 = call "Write Reset.vi"("error in"=w554, "Reset Arguments"=T38."Reset counter (all)", "MB_TCP session in"=w559) -> ("error out"=w553:errorcluster, "MB session out"=w557:refnum<class "MB_Master_TCP.lvclass">)  [unwired: 7 in]
              n102 = Bundle By Name(cluster=w558, "MB_TCP session"=w557) -> (w556:T3)
            }
            n103 = Bundle By Name(cluster=w549, "Flexi-Flow Devices"=w546) -> (w548:T2)
          }
          frame "Read Device User Tag" {
            # "Reads the user tag of the device."
            n104 = Variant To Data(error in=w574, type=T32 {"Device"=enum."Hydrogen Inlet"} ("Read Device User Tag Argument"), Variant=w573) -> (data=w571:T32, error out=w567:errorcluster)
            n105 = Unbundle By Name(w571) -> ("Device"=w569:T15)
            n106 = call "Get Device Modbus TCP Session.vi"("Device"=w569, "Data Cluster In"=w568) -> ("Device State"=w562:T3, "MB_TCP session"=w564:refnum<class "MB_Master_TCP.lvclass">, "Data Cluster Out"=w570:T2)  [unwired: 7 in]
            n107 = call "Read User Tag.vi"("error in"=w567, "MB_TCP session in"=w564) -> ("error out"=w566:errorcluster, "Value"=w560:string, "MB session out"=w565:refnum<class "MB_Master_TCP.lvclass">)  [unwired: 7 in]
            n108 = Bundle By Name(cluster=w562, "User Tag"=w560) -> (w561:T3)
            n109 = call "Update Device.vi"("Device"=w569, "Device State"=w561, "MB_TCP session"=w565, "Data Cluster"=w570) -> ("Data Cluster Out"=w563:T2)  [unwired: 7 in]
          }
          frame "Set Device User Tag" {
            # "Sets the device user tag."
            n110 = Variant To Data(error in=w588, type=T33 {"Device"=enum."Hydrogen Inlet", "User Tag"=""} ("Set Device User Tag Argument"), Variant=w587) -> (data=w585:T33, error out=w579:errorcluster)
            n111 = Unbundle By Name(w585) -> ("Device"=w580:T15, "User Tag"=w575:string)
            n112 = call "Get Device Modbus TCP Session.vi"("Device"=w580, "Data Cluster In"=w582) -> ("Device State"=w583:T3, "MB_TCP session"=w577:refnum<class "MB_Master_TCP.lvclass">, "Data Cluster Out"=w584:T2)  [unwired: 7 in]
            n113 = call "Write User Tag.vi"("error in"=w579, "Label"=w575, "MB_TCP session in"=w577) -> ("error out"=w578:errorcluster, "MB session out"=w576:refnum<class "MB_Master_TCP.lvclass">)  [unwired: 7 in]
            n114 = call "Update Device.vi"("Device"=w580, "Device State"=w583, "MB_TCP session"=w576, "Data Cluster"=w584) -> ("Data Cluster Out"=w581:T2)  [unwired: 7 in]
          }
          frame "Read Counter Unit" {
            # "#CodeNeeded\n1. Configure this Message Case for handling the \"Read Counter Unit\" message.\n2. Delete or edit this label when done."
            # "Reads the counter unit."
            n115 = Variant To Data(error in=w602, type=T34 {"Device"=enum."Hydrogen Inlet"} ("Read Counter Unit Argument"), Variant=w601) -> (data=w599:T34, error out=w591:errorcluster)
            n116 = Unbundle By Name(w599) -> ("Device"=w594:T15)
            n117 = call "Get Device Modbus TCP Session.vi"("Device"=w594, "Data Cluster In"=w596) -> ("Device State"=w597:T3, "MB_TCP session"=w593:refnum<class "MB_Master_TCP.lvclass">, "Data Cluster Out"=w598:T2)  [unwired: 7 in]
            n118 = call "Read Counter Unit.vi"("error in"=w591, "MB_TCP session in"=w593) -> ("error out"=w590:errorcluster, "Value"=→"Counter Unit":string, "MB session out"=w592:refnum<class "MB_Master_TCP.lvclass">)  [unwired: 7 in]
            n119 = call "Update Device.vi"("Device"=w594, "Device State"=w597, "MB_TCP session"=w592, "Data Cluster"=w598) -> ("Data Cluster Out"=w595:T2)  [unwired: 7 in]
          }
          frame "Set Control Mode" {
            # "Sets the flexi-flow control mode."
            n120 = Variant To Data(error in=w617, type=T35 {"Device"=enum."Hydrogen Inlet", "Control Mode"=0} ("Set Control Mode Argument"), Variant=w616) -> (data=w614:T35, error out=w605:errorcluster)
            n121 = Unbundle By Name(w614) -> ("Device"=w610:T15, "Control Mode"=w603:T6)
            n122 = call "Get Device Modbus TCP Session.vi"("Device"=w610, "Data Cluster In"=w609) -> ("Device State"=w612:T3, "MB_TCP session"=w607:refnum<class "MB_Master_TCP.lvclass">, "Data Cluster Out"=w613:T2)  [unwired: 7 in]
            n123 = call "Write Control Mode.vi"("error in"=w605, "Control Mode"=w603, "MB_TCP session in"=w607) -> ("error out"=w604:errorcluster, "MB session out"=w606:refnum<class "MB_Master_TCP.lvclass">)  [unwired: 7 in]
            n124 = Bundle By Name(cluster=w612, "Control State.Control Mode"=w603) -> (w611:T3)
            n125 = call "Update Device.vi"("Device"=w610, "Device State"=w611, "MB_TCP session"=w606, "Data Cluster"=w613) -> ("Data Cluster Out"=w608:T2)  [unwired: 7 in]
          }
          frame "Get Device Configuration" {
            # "Gets the device configuration."
            n126 = Variant To Data(error in=w631, type=T36 {"Device"=enum."Hydrogen Inlet"} ("Get Device Configuration Argument"), Variant=w630) -> (data=w626:T36, error out=w619:errorcluster)
            n127 = Unbundle By Name(w626) -> ("Device"=w627:T15)
            n128 = call "Get Device Modbus TCP Session.vi"("Device"=w627, "Data Cluster In"=w625) -> ("Device State"=w621:T3, "MB_TCP session"=w623:refnum<class "MB_Master_TCP.lvclass">, "Data Cluster Out"=w628:T2)  [unwired: 7 in]
            n129 = call "Get Device Configuration--SubVI.vi"("error in (no error)"=w619, "Device State in"=w621, "MB_Master_TCP in"=w623) -> ("error out"=w618:errorcluster, "Device State out"=w620:T3, "MB_Master_TCP out"=w622:refnum<class "MB_Master_TCP.lvclass">)  [unwired: 6 in]
            n130 = call "Update Device.vi"("Device"=w627, "Device State"=w620, "MB_TCP session"=w622, "Data Cluster"=w628) -> ("Data Cluster Out"=w624:T2)  [unwired: 7 in]
          }
          frame "---Copy This Frame---" {
            # "Duplicate this frame when creating new messages.  Change this comment in the duplicated frame to describe this message."
            n131 = Merge Errors(w634) -> (w633:errorcluster)
          }
          frame "--- Exit and Error Handling---" {
            # "Separator - The following cases handle errors and exit messages."
            n132 = Merge Errors(w637) -> (w636:errorcluster)
          }
          frame "Simulate MHL Error" {
            # "Simulate an error occurring at the MHL"
            n133 = call "Module Name--constant.vi"() -> ("Module Name"=w640:string)  [unwired: 11 in]
            n134 = xnode "Error Ring"("parameter 0"=w640) -> ("error out"=w639:errorcluster)
            n135 = Merge Errors(w642, w639) -> (w641:errorcluster)
          }
          frame "Error" {
            # "#CodeRecommended - If you ever change the name of this \"Error\" message, you'll need to update the name in the Check Loop Error.vi as well."
            # "#CodeRecommended - If the module is running in standalone mode (External Launch = FALSE), this code will pop up an error dialog and call the 'Exit' message if an error occurs. Add more fine-grained error handling here."
            # "Error - Check the error message data and respond accordingly. This message is sent by the \"Error Handler\" VIs at the end of each loop in this application."
            n136 = property class="Module Admin"(reference=w653) -> ("Accessors:External Launch"=w652:bool)  [unwired: 1 in, 2 out]
            n137 = Variant To Data(error in=w659, type=errorcluster {"status"=FALSE, "code"=0, "source"=""} ("error constant"), Variant=w658) -> (data=w660:errorcluster, error out=w656:errorcluster)
            n138 = call "Error Reported.vi"("Error"=w660) -> ()  [unwired: 10 in, 1 out]
            n139 = case shown="False" w652 {
              tunnel: [w665 _] -> w655
              tunnel: w654 -> [w664 _]
              tunnel: w660 -> [w661 _]
              frame False {
                # "If the module is running standalone, then pop up an error dialog and call the \"Exit\" message."
                n140 = call <vilib>:"Simple Error Handler.vi"("error in (no error)"=w661) -> ()  [unwired: 4 in, 5 out]
                n141 = call-poly <vilib>:"Delacor_lib_QMH_Enqueue Message (poly).vi"("Priority Message? (F)"=TRUE, "Message"="Exit", "Message Queue in"=w664) -> ("error out"=w665:errorcluster)  [unwired: 7 in, 1 out]
              }
              frame True {
                # "If the module was launched externally, calling the Error Reported broadcast VI is the only action performed by the \"Error\" message. The module's caller can then process the error appropriately."
              }
            }
            n142 = Merge Errors(w656, w655) -> (w651:errorcluster)
            n143 = local write "error out"(w651) -> ()
          }
          frame "Confirm Quit" {
            # "#CodeNeeded - If you want to provide an \"Are you sure\" dialog (or some other notification) before the application exits, place that code here. This message is typically sent from a Panel Close? event."
            # "Confirm Quit - Message that can confirm whether or not the user wants to exit the application."
            n144 = call-poly <vilib>:"Delacor_lib_QMH_Enqueue Message (poly).vi"("Priority Message? (F)"=TRUE, "error in"=w672, "Message"="Exit", "Message Queue in"=w669) -> ("error out"=w670:errorcluster)  [unwired: 6 in, 1 out]
            n145 = Merge Errors(w670) -> (w671:errorcluster)
          }
          frame "Exit" {
            w681 = 91  # 91: not all Exit messages will have an argument
            w686 = TRUE  # Stop the VI
            # "Release the message queue reference"
            # "Exit - Exit the application."
            n146 = Variant To Data(error in=w689, type=T13 {"Origin"="", "Exit via Stop Module Req?"=FALSE, "Wait for Module to stop?"=FALSE} ("Stop Argument"), Variant=w683) -> (data=w679:T13, error out=w682:errorcluster)
            n147 = call <vilib>:"Clear Errors.vi"("error in (no error)"=w682, "specific error code to clear (0: all)"=w681) -> ("error out"=w688:errorcluster)  [unwired: 4 in, 1 out]
            n148 = Unbundle By Name(w675) -> ("MB_TCP_sessions"=w674:refnum<class "MB_Master_TCP.lvclass">[])
            n149 = call-dynamic "Delacor_lib_QMH_Release Message Queue.vi"("error in"=w688, "Message Queue"=w687) -> ("error out"=w685:errorcluster)  [unwired: 9 in]
            n150 = for {
              tunnel: [w691] -> w676
              tunnel: w674 -> [w690] mode=indexing
              n151 = call "Modbus TCP Close.vi"("MB session in"=w690) -> ("error out"=w691:errorcluster)  [unwired: 10 in]
            }
            n152 = call "Handle Exit.vi"("Stop Argument"=w679, "Admin in"=w678) -> ("error out"=w677:errorcluster)  [unwired: 8 in, 1 out]
            n153 = call "Sleep Modbus Polling Helper Loop.vi"() -> ("error out"=w673:errorcluster)  [unwired: 11 in]
            n154 = Merge Errors(w673, w677, w676, w685) -> (w684:errorcluster)
          }
          frame Default {
            # "'Default' case only runs if there is a message that isn't defined in any of the other cases.  Output a programming error."
            n155 = call "Module Name--constant.vi"() -> ("Module Name"=w693:string)  [unwired: 11 in]
            n156 = xnode "Error Ring"("parameter 0"=w694, "parameter 1"=w693) -> ("error out"=w695:errorcluster)
          }
        }
        "Data Cluster" <- w320
        n157 = call-dynamic "Delacor_lib_QMH_Error Handler - Message Handling Loop.vi"("error in"=w331, "Message Queue in"=w323) -> ("dup error in"=w322:errorcluster)  [unwired: 8 in, 1 out]
      }
      n158 = while {
        tunnel: w36 -> [w87]
        shift-right: [w85] -> w48
        shift-left: w46 -> [w86]
        tunnel: [w81] -> w45
        tunnel: w43 -> [w80]
        tunnel: w42 -> [w79]
        shift-right: [w77] -> w40
        shift-left: w41 -> [w78]
        stop <- w83 stop-if-true
        # "Event Handling Loop"
        n159 = event "DQMH_EVENT_MAIN" shown="[27] <FlexiFlowInterfaceCH2 Request Events.Get Device Configuration>: User Event" {
          selector: w86 -> [_ _ _ _ _ _ _ _ _ _ _ _ _ _ _ _ _ _ _ _ _ _ _ _ _ _ _ _]
          dyn-events: [_ _ _ _ _ _ _ _ _ _ _ _ _ _ _ _ _ _ _ _ _ _ _ _ _ _ _ _] -> w85
          timeout: _ -> [_ _ _ _ _ _ _ _ _ _ _ _ _ _ _ _ _ _ _ _ _ _ _ _ _ _ _ _]
          tunnel: [_ _ _ _ _ _ TRUE ("Discard?") _ _ _ _ _ _ _ _ _ _ _ _ _ _ _ _ _ _ _ _ _] -> w83
          tunnel: w87 -> [w91 w103 w107 w110 w114 w119 w131 w141 w148 w165 w173 w182 w190 w198 w206 w215 w224 w233 w242 w251 w260 w269 w277 w285 w294 w302 w311 w319]
          tunnel: [w90 w100 w105 _ w113 w116 w125 w137 w147 w158 w166 w176 w183 w191 w199 w207 w216 w227 w234 w243 w252 w263 w270 w278 w286 w296 w303 w312] -> w84
          tunnel: [w91 w102 w107 w110 w114 w118 w130 w141 w146 w163 w171 w180 w188 w196 w204 w213 w222 w231 w240 w249 w258 w267 w275 w283 w292 w300 w309 w317] -> w82
          tunnel: w80 -> [_ _ _ _ _ _ _ _ w145 _ _ _ _ _ _ _ _ _ _ _ _ _ _ _ _ _ _ _]
          tunnel: w79 -> [_ _ _ _ _ _ _ w136 _ _ _ _ _ _ _ _ _ _ _ _ _ _ _ _ _ _ _ _]
          tunnel: w78 -> [w88 w99 w106 w109 w111 w115 w120 w140 w143 w164 w172 w181 w189 w197 w205 w214 w223 w232 w241 w250 w259 w268 w276 w284 w293 w301 w310 w318]
          tunnel: [w88 w99 w106 w109 w111 w115 w120 w135 w142 w164 w172 w181 w189 w197 w205 w214 w223 w232 w241 w250 w259 w268 w276 w284 w293 w301 w310 w318] -> w77
          event "Simulate EHL Error": Value Change {
            # "This case simulates an error being generated at the EHL"
            n160 = event-data() -> ()  [unwired: 1 in, 1 out]
            n161 = call "Module Name--constant.vi"() -> ("Module Name"=w89:string)  [unwired: 11 in]
            n162 = xnode "Error Ring"("parameter 0"=w89) -> ("error out"=w90:errorcluster)
          }
          event "Simulate MHL Error": Value Change {
            # "This case simulates an error being generated at the EHL"
            n163 = event-data() -> ()  [unwired: 1 in, 1 out]
            n164 = call-poly <vilib>:"Delacor_lib_QMH_Enqueue Message (poly).vi"("Message"="Simulate MHL Error", "Message Queue in"=w103) -> ("error out"=w100:errorcluster, "Message Queue out"=w102:refnum<class "Delacor_lib_QMH_Message Queue.lvclass">)  [unwired: 8 in]
          }
          event User Event {
            # "Another Module called the \"Show Panel\" API Method."
            n165 = event-data() -> ()  [unwired: 1 in, 1 out]
            n166 = call <vilib>:"Show.vi"("Panel in"=w106) -> ("Error Out"=w105:errorcluster)  [unwired: 10 in]
            n167 = call "Status Updated.vi"("Status"="Panel shown." ("format string")) -> ()  [unwired: 10 in, 1 out]
          }
          event User Event {
            # "Another Module called the \"Hide Panel\" API Method."
            n168 = event-data() -> ()  [unwired: 1 in, 1 out]
            n169 = call <vilib>:"Hide.vi"("Panel In"=w109) -> ()  [unwired: 10 in, 1 out]
            n170 = call "Status Updated.vi"("Status"="Panel hidden." ("format string")) -> ()  [unwired: 10 in, 1 out]
          }
          event User Event {
            # "Another Module called the \"Get Module Execution Status\" API Method."
            n171 = event-data() -> ()  [unwired: 1 in, 1 out]
            n172 = call "Update Module Execution Status.vi"("Running?"=TRUE) -> ("error out"=w113:errorcluster)  [unwired: 10 in]
          }
          event User Event {
            # "Another Module called the \"Show Diagram\" API Method."
            n173 = event-data() -> ()  [unwired: 1 in, 1 out]
            n174 = call-poly <vilib>:"Delacor_lib_QMH_Enqueue Message (poly).vi"("Message"="Show Diagram", "Message Queue in"=w119) -> ("error out"=w116:errorcluster, "Message Queue out"=w118:refnum<class "Delacor_lib_QMH_Message Queue.lvclass">)  [unwired: 8 in]
          }
          event User Event {
            # "The Stop Module Event can get fired from the Exit message in the MHL. The queue gets destroyed in that case. If the queue no longer exists, the Enqueue Exit as a priority message will return error 1. It is safe to ignore, because the module is already exiting."
            # "Another Module called the \"Stop Module\" API Method  or the Message Handling Loop below."
            n175 = event-data() -> ("Origin"=w129:string, "Exit via Stop Module Req?"=w123:bool, "Wait for Module to stop?"=w122:bool)  [unwired: 1 in]
            n176 = call <vilib>:"Hide.vi"("Panel In"=w120) -> ()  [unwired: 10 in, 1 out]
            n177 = local write "Status"(w129) -> ()
            n178 = Bundle By Name(cluster=T13 {"Origin"="", "Exit via Stop Module Req?"=FALSE, "Wait for Module to stop?"=FALSE} ("Stop Argument"), "Exit via Stop Module Req?"=w123, "Wait for Module to stop?"=w122) -> (w121:T13)
            n179 = call-poly <vilib>:"Delacor_lib_QMH_Enqueue Message (poly).vi"("Priority Message? (F)"=TRUE, "Message Data"=w121, "Message"="Exit", "Message Queue in"=w131) -> ("error out"=w126:errorcluster, "Message Queue out"=w130:refnum<class "Delacor_lib_QMH_Message Queue.lvclass">)  [unwired: 6 in]
            n180 = call <vilib>:"Clear Errors.vi"("error in (no error)"=w126, "specific error code to clear (0: all)"=1) -> ("error out"=w125:errorcluster)  [unwired: 4 in, 1 out]
          }
          event User Event {
            # "Another Module called the \"Change Panel\" API Method."
            n181 = event-data() -> ("New Panel"=w139:refnum<class "Panel.lvclass">)  [unwired: 1 in]
            n182 = call-dynamic <vilib>:"Close.vi"("Panel In"=w140) -> ("Error Out"=w138:errorcluster)  [unwired: 10 in]
            n183 = call <vilib>:"Initialize.vi"("error in (no error)"=w138, "My Helper in"=w136, "Panel In"=w139) -> ("error out"=w137:errorcluster, "Panel Out"=w135:refnum<class "Panel.lvclass">)  [unwired: 6 in, 1 out]
            n184 = call "Status Updated.vi"("Status"="Panel changed.") -> ()  [unwired: 10 in, 1 out]
          }
          event Panel Close? {
            w149 = TRUE  # Discard the event so the 'Confirm Quit' message has a chance to run.
            # "If launched externally, closing the panel doesn't quit the VI."
            # "Send the 'Confirm Quit' message if the user closes the panel of the VI."
            n185 = event-data() -> ()  [unwired: 1 in, 1 out]
            n186 = property class="Module Admin"(reference=w145) -> ("Accessors:External Launch"=w144:bool)  [unwired: 1 in, 2 out]
            n187 = case shown="True" w144 {
              tunnel: w148 -> [w154 w157]
              tunnel: [w153 w155] -> w147
              tunnel: [w152 w157] -> w146
              tunnel: w143 -> [w150 w156]
              tunnel: [w150 w156] -> w142
              frame False {
                n188 = call-poly <vilib>:"Delacor_lib_QMH_Enqueue Message (poly).vi"("Message"="Confirm Quit", "Message Queue in"=w154) -> ("error out"=w153:errorcluster, "Message Queue out"=w152:refnum<class "Delacor_lib_QMH_Message Queue.lvclass">)  [unwired: 8 in]
              }
              frame True {
                n189 = call <vilib>:"Hide.vi"("Panel In"=w156) -> ("Error Out"=w155:errorcluster)  [unwired: 10 in]
              }
            }
            n190 = event-data("Discard?"=w149) -> ()  [unwired: 1 in, 1 out]
          }
          event User Event {
            # "Another Module called the \"Initialise Modbus Connections\" API Method."
            n191 = event-data() -> ("Boolean"=w159:bool)  [unwired: 1 in]
            n192 = Bundle(cluster=T12 {"Boolean"=FALSE} ("Initialise Modbus Connections Argument"), "Boolean"=w159) -> (w160:T12)
            n193 = call-poly <vilib>:"Delacor_lib_QMH_Enqueue Message (poly).vi"("Message Data"=w160, "Message"="Initialise Modbus Connections", "Message Queue in"=w165) -> ("error out"=w158:errorcluster, "Message Queue out"=w163:refnum<class "Delacor_lib_QMH_Message Queue.lvclass">)  [unwired: 7 in]
          }
          event User Event {
            # "Another Module called the \"Read Device State\" API Method."
            n194 = event-data() -> ("Device"=w167:T15)  [unwired: 1 in]
            n195 = Bundle(cluster=T14 {"Device"=enum."Hydrogen Inlet"} ("Read Device State Argument"), "Device"=w167) -> (w168:T14)
            n196 = call-poly <vilib>:"Delacor_lib_QMH_Enqueue Message (poly).vi"("Message Data"=w168, "Message"="Read Measure", "Message Queue in"=w173) -> ("error out"=w166:errorcluster, "Message Queue out"=w171:refnum<class "Delacor_lib_QMH_Message Queue.lvclass">)  [unwired: 7 in]
          }
          event User Event {
            # "Another Module called the \"Set Modbus Configuration\" API Method."
            n197 = event-data() -> ("Device"=w174:T15, "Modbus TCP Connection"=w175:T1)  [unwired: 1 in]
            n198 = Bundle(cluster=T16 {"Device"=enum."Hydrogen Inlet", "Modbus TCP Connection"={"Label"="", "Slave ID (255)"=255, "IP Address"="", "Port (502)"=502, "Timeout (10000)"=10000}} ("Set Modbus Configuration Argument"), "Device"=w174, "Modbus TCP Connection"=w175) -> (w177:T16)
            n199 = call-poly <vilib>:"Delacor_lib_QMH_Enqueue Message (poly).vi"("Message Data"=w177, "Message"="Set Modbus Configuration", "Message Queue in"=w182) -> ("error out"=w176:errorcluster, "Message Queue out"=w180:refnum<class "Delacor_lib_QMH_Message Queue.lvclass">)  [unwired: 7 in]
          }
          event User Event {
            # "Another Module called the \"Wink Devices\" API Method."
            n200 = event-data() -> ("Boolean"=w184:bool)  [unwired: 1 in]
            n201 = Bundle(cluster=T17 {"Boolean"=FALSE} ("Wink Devices Argument"), "Boolean"=w184) -> (w185:T17)
            n202 = call-poly <vilib>:"Delacor_lib_QMH_Enqueue Message (poly).vi"("Message Data"=w185, "Message"="Wink Devices", "Message Queue in"=w190) -> ("error out"=w183:errorcluster, "Message Queue out"=w188:refnum<class "Delacor_lib_QMH_Message Queue.lvclass">)  [unwired: 7 in]
          }
          event User Event {
            # "Another Module called the \"Read All FlexiFlow Device States\" API Method."
            n203 = event-data() -> ("Boolean"=w192:bool)  [unwired: 1 in]
            n204 = Bundle(cluster=T18 {"Boolean"=FALSE} ("Read All FlexiFlow Device States Argument"), "Boolean"=w192) -> (w193:T18)
            n205 = call-poly <vilib>:"Delacor_lib_QMH_Enqueue Message (poly).vi"("Message Data"=w193, "Message"="Read All FlexiFlow Device States", "Message Queue in"=w198) -> ("error out"=w191:errorcluster, "Message Queue out"=w196:refnum<class "Delacor_lib_QMH_Message Queue.lvclass">)  [unwired: 7 in]
          }
          event User Event {
            # "Another Module called the \"Wink Device\" API Method."
            n206 = event-data() -> ("Device"=w200:T15)  [unwired: 1 in]
            n207 = Bundle(cluster=T19 {"Device"=enum."Hydrogen Inlet"} ("Wink Device Argument"), "Device"=w200) -> (w201:T19)
            n208 = call-poly <vilib>:"Delacor_lib_QMH_Enqueue Message (poly).vi"("Message Data"=w201, "Message"="Wink Device", "Message Queue in"=w206) -> ("error out"=w199:errorcluster, "Message Queue out"=w204:refnum<class "Delacor_lib_QMH_Message Queue.lvclass">)  [unwired: 7 in]
          }
          event User Event {
            # "Another Module called the \"Set Control Function\" API Method."
            n209 = event-data() -> ("Device"=w209:T15, "Function"=w208:T7)  [unwired: 1 in]
            n210 = Bundle(cluster=T20 {"Device"=enum."Hydrogen Inlet", "Function"=enum."Flow"} ("Set Control Function Argument"), "Device"=w209, "Function"=w208) -> (w210:T20)
            n211 = call-poly <vilib>:"Delacor_lib_QMH_Enqueue Message (poly).vi"("Message Data"=w210, "Message"="Set Control Function", "Message Queue in"=w215) -> ("error out"=w207:errorcluster, "Message Queue out"=w213:refnum<class "Delacor_lib_QMH_Message Queue.lvclass">)  [unwired: 7 in]
          }
          event User Event {
            # "Another Module called the \"Set Control Value SP\" API Method."
            n212 = event-data() -> ("Device"=w218:T15, "Setpoint Value"=w217:dbl)  [unwired: 1 in]
            n213 = Bundle(cluster=T21 {"Device"=enum."Hydrogen Inlet", "Setpoint Value"=0.0} ("Set Control Value SP Argument"), "Device"=w218, "Setpoint Value"=w217) -> (w219:T21)
            n214 = call-poly <vilib>:"Delacor_lib_QMH_Enqueue Message (poly).vi"("Message Data"=w219, "Message"="Set Flow Setpoint", "Message Queue in"=w224) -> ("error out"=w216:errorcluster, "Message Queue out"=w222:refnum<class "Delacor_lib_QMH_Message Queue.lvclass">)  [unwired: 7 in]
          }
          event User Event {
            # "Another Module called the \"Set Backpressure Setpoint\" API Method."
            n215 = event-data() -> ("Device"=w225:T15, "Backpressure SP"=w226:dbl)  [unwired: 1 in]
            n216 = Bundle(cluster=T22 {"Device"=enum."Cathode Outlet", "Backpressure SP"=0.0} ("Set Backpressure Setpoint Argument"), "Device"=w225, "Backpressure SP"=w226) -> (w228:T22)
            n217 = call-poly <vilib>:"Delacor_lib_QMH_Enqueue Message (poly).vi"("Message Data"=w228, "Message"="Set Backpressure Setpoint", "Message Queue in"=w233) -> ("error out"=w227:errorcluster, "Message Queue out"=w231:refnum<class "Delacor_lib_QMH_Message Queue.lvclass">)  [unwired: 7 in]
          }
          event User Event {
            # "Another Module called the \"Set Forward Pressure SP\" API Method."
            n218 = event-data() -> ("Device"=w236:T15, "Pressure SP"=w235:dbl)  [unwired: 1 in]
            n219 = Bundle(cluster=T23 {"Device"=enum."Hydrogen Inlet", "Pressure SP"=0.0} ("Set Forward Pressure SP Argument"), "Device"=w236, "Pressure SP"=w235) -> (w237:T23)
            n220 = call-poly <vilib>:"Delacor_lib_QMH_Enqueue Message (poly).vi"("Message Data"=w237, "Message"="Set Forward Pressure SP", "Message Queue in"=w242) -> ("error out"=w234:errorcluster, "Message Queue out"=w240:refnum<class "Delacor_lib_QMH_Message Queue.lvclass">)  [unwired: 7 in]
          }
          event User Event {
            # "Another Module called the \"Set Flow Capacity Unit\" API Method."
            n221 = event-data() -> ("Device"=w245:T15, "Standard Volume Flow"=w244:T25)  [unwired: 1 in]
            n222 = Bundle(cluster=T24 {"Device"=enum."Hydrogen Inlet", "Standard Volume Flow"=0} ("Set Flow Capacity Unit Argument"), "Device"=w245, "Standard Volume Flow"=w244) -> (w246:T24)
            n223 = call-poly <vilib>:"Delacor_lib_QMH_Enqueue Message (poly).vi"("Message Data"=w246, "Message"="Set Flow Capacity Unit", "Message Queue in"=w251) -> ("error out"=w243:errorcluster, "Message Queue out"=w249:refnum<class "Delacor_lib_QMH_Message Queue.lvclass">)  [unwired: 7 in]
          }
          event User Event {
            # "Another Module called the \"Set Setpoint Slope\" API Method."
            n224 = event-data() -> ("Setpoint Slope"=w254:u16, "Device"=w253:T15)  [unwired: 1 in]
            n225 = Bundle(cluster=T26 {"Setpoint Slope"=0, "Device"=enum."Hydrogen Inlet"} ("Set Setpoint Slope Argument"), "Setpoint Slope"=w254, "Device"=w253) -> (w255:T26)
            n226 = call-poly <vilib>:"Delacor_lib_QMH_Enqueue Message (poly).vi"("Message Data"=w255, "Message"="Set Setpoint Slope", "Message Queue in"=w260) -> ("error out"=w252:errorcluster, "Message Queue out"=w258:refnum<class "Delacor_lib_QMH_Message Queue.lvclass">)  [unwired: 7 in]
          }
          event User Event {
            # "Another Module called the \"Set Counter Settings\" API Method."
            n227 = event-data() -> ("Device"=w262:T15, "Counter Settings"=w261:T28)  [unwired: 1 in]
            n228 = Bundle(cluster=T27 {"Device"=enum."Hydrogen Inlet", "Counter Settings"={"Counter Setpoint Mode"=enum."No setpoint change (default)", "Counter Limit"=0.0, "Unit"="ls", "Counter Mode"=enum."Counter off (default)", "Counter New Setpoint"=0}} ("Set Counter Settings Argument"), "Device"=w262, "Counter Settings"=w261) -> (w264:T27)
            n229 = call-poly <vilib>:"Delacor_lib_QMH_Enqueue Message (poly).vi"("Message Data"=w264, "Message"="Set Counter Settings", "Message Queue in"=w269) -> ("error out"=w263:errorcluster, "Message Queue out"=w267:refnum<class "Delacor_lib_QMH_Message Queue.lvclass">)  [unwired: 7 in]
          }
          event User Event {
            # "Another Module called the \"Reset All Device Counters\" API Method."
            n230 = event-data() -> ("Boolean"=w271:bool)  [unwired: 1 in]
            n231 = Bundle(cluster=T31 {"Boolean"=FALSE} ("Reset All Device Counters Argument"), "Boolean"=w271) -> (w272:T31)
            n232 = call-poly <vilib>:"Delacor_lib_QMH_Enqueue Message (poly).vi"("Message Data"=w272, "Message"="Reset All Device Counters", "Message Queue in"=w277) -> ("error out"=w270:errorcluster, "Message Queue out"=w275:refnum<class "Delacor_lib_QMH_Message Queue.lvclass">)  [unwired: 7 in]
          }
          event User Event {
            # "Another Module called the \"Read Device User Tag\" API Method."
            n233 = event-data() -> ("Device"=w279:T15)  [unwired: 1 in]
            n234 = Bundle(cluster=T32 {"Device"=enum."Hydrogen Inlet"} ("Read Device User Tag Argument"), "Device"=w279) -> (w280:T32)
            n235 = call-poly <vilib>:"Delacor_lib_QMH_Enqueue Message (poly).vi"("Message Data"=w280, "Message"="Read Device User Tag", "Message Queue in"=w285) -> ("error out"=w278:errorcluster, "Message Queue out"=w283:refnum<class "Delacor_lib_QMH_Message Queue.lvclass">)  [unwired: 7 in]
          }
          event User Event {
            # "Another Module called the \"Set Device User Tag\" API Method."
            n236 = event-data() -> ("Device"=w288:T15, "User Tag"=w287:string)  [unwired: 1 in]
            n237 = Bundle(cluster=T33 {"Device"=enum."Hydrogen Inlet", "User Tag"=""} ("Set Device User Tag Argument"), "Device"=w288, "User Tag"=w287) -> (w289:T33)
            n238 = call-poly <vilib>:"Delacor_lib_QMH_Enqueue Message (poly).vi"("Message Data"=w289, "Message"="Set Device User Tag", "Message Queue in"=w294) -> ("error out"=w286:errorcluster, "Message Queue out"=w292:refnum<class "Delacor_lib_QMH_Message Queue.lvclass">)  [unwired: 7 in]
          }
          event User Event {
            # "Another Module called the \"Read Counter Unit\" API Method."
            n239 = event-data() -> ("Device"=w295:T15)  [unwired: 1 in]
            n240 = Bundle(cluster=T34 {"Device"=enum."Hydrogen Inlet"} ("Read Counter Unit Argument"), "Device"=w295) -> (w297:T34)
            n241 = call-poly <vilib>:"Delacor_lib_QMH_Enqueue Message (poly).vi"("Message Data"=w297, "Message"="Read Counter Unit", "Message Queue in"=w302) -> ("error out"=w296:errorcluster, "Message Queue out"=w300:refnum<class "Delacor_lib_QMH_Message Queue.lvclass">)  [unwired: 7 in]
          }
          event User Event {
            # "Another Module called the \"Set Control Mode\" API Method."
            n242 = event-data() -> ("Device"=w305:T15, "Control Mode"=w304:T6)  [unwired: 1 in]
            n243 = Bundle(cluster=T35 {"Device"=enum."Hydrogen Inlet", "Control Mode"=0} ("Set Control Mode Argument"), "Device"=w305, "Control Mode"=w304) -> (w306:T35)
            n244 = call-poly <vilib>:"Delacor_lib_QMH_Enqueue Message (poly).vi"("Message Data"=w306, "Message"="Set Control Mode", "Message Queue in"=w311) -> ("error out"=w303:errorcluster, "Message Queue out"=w309:refnum<class "Delacor_lib_QMH_Message Queue.lvclass">)  [unwired: 7 in]
          }
          event User Event {
            # "Another Module called the \"Get Device Configuration\" API Method."
            n245 = event-data() -> ("Device"=w313:T15)  [unwired: 1 in]
            n246 = Bundle(cluster=T36 {"Device"=enum."Hydrogen Inlet"} ("Get Device Configuration Argument"), "Device"=w313) -> (w314:T36)
            n247 = call-poly <vilib>:"Delacor_lib_QMH_Enqueue Message (poly).vi"("Message Data"=w314, "Message"="Get Device Configuration", "Message Queue in"=w319) -> ("error out"=w312:errorcluster, "Message Queue out"=w317:refnum<class "Delacor_lib_QMH_Message Queue.lvclass">)  [unwired: 7 in]
          }
        }
        n248 = call-dynamic "Delacor_lib_QMH_Error Handler - Event Handling Loop.vi"("error in"=w84, "Message Queue in"=w82) -> ("dup error in"=w81:errorcluster)  [unwired: 8 in, 1 out]
      }
      n249 = while {
        shift-right: [w67] -> _
        shift-left: -1 -> [w68]
        tunnel: w38 -> [w66]
        tunnel: w36 -> [w64]
        stop <- w65 stop-if-true
        n250 = event shown="[0] Timeout" {
          selector: w66 -> [_ _ _ _]
          dyn-events: _ -> [_ _ _ _]
          timeout: w68 -> [_ _ _ _]
          tunnel: w68 -> [w72 _ _ _]
          tunnel: [w72 1000 -1 -1] -> w67
          tunnel: [_ _ _ TRUE] -> w65
          tunnel: w64 -> [w69 _ _ _]
          tunnel: [w70 _ _ _] -> _
          event Timeout {
            n251 = event-data() -> ()  [unwired: 1 in, 3 out]
            n252 = call-poly <vilib>:"Delacor_lib_QMH_Enqueue Message (poly).vi"("Message"="Read All FlexiFlow Device States", "Message Queue in"=w69) -> ("error out"=w70:errorcluster)  [unwired: 8 in, 1 out]
          }
          event User Event {
            n253 = event-data() -> ()  [unwired: 1 in, 3 out]
          }
          event User Event {
            n254 = event-data() -> ()  [unwired: 1 in, 3 out]
          }
          event User Event {
            n255 = event-data() -> ()  [unwired: 1 in, 3 out]
          }
        }
      }
      n256 = while {
        shift-right: [w53] -> _
        shift-left: -1 -> [w54]
        tunnel: w35 -> [w52]
        tunnel: w36 -> [w50]
        stop <- w51 stop-if-true
        # "Connection Helper Loop"
        n257 = event shown="[2] <Sleep Connection Helper Loop>: User Event" {
          selector: w52 -> [_ _ _ _]
          dyn-events: _ -> [_ _ _ _]
          timeout: w54 -> [_ _ _ _]
          tunnel: w54 -> [w59 _ _ _]
          tunnel: [w59 1000 -1 -1] -> w53
          tunnel: [_ _ _ TRUE] -> w51
          tunnel: w50 -> [w56 _ _ _]
          tunnel: [w57 _ _ _] -> _
          event Timeout {
            n258 = event-data() -> ()  [unwired: 1 in, 3 out]
            n259 = call-poly <vilib>:"Delacor_lib_QMH_Enqueue Message (poly).vi"("Message Data"=T12 {"Boolean"=FALSE} ("Initialise Modbus Connections Argument"), "Message"="Initialise Modbus Connections", "Message Queue in"=w56) -> ("error out"=w57:errorcluster)  [unwired: 7 in, 1 out]
          }
          event User Event {
            n260 = event-data() -> ()  [unwired: 1 in, 5 out]
          }
          event User Event {
            n261 = event-data() -> ()  [unwired: 1 in, 5 out]
          }
          event User Event {
            n262 = event-data() -> ()  [unwired: 1 in, 3 out]
          }
        }
      }
    }
    frame Error {
      # "Synchronize Caller Events.vi will inform Start Module.vi that the module has launched and will let the code calling Start Module.vi register for broadcasts and would permit the caller receive the broadcast that an error occurred at launch time."
      n263 = call "Synchronize Caller Events.vi"("Singleton Module Admin in"=w708) -> ("error out"=w705:errorcluster)  [unwired: 9 in, 1 out]
      n264 = call "Module Name--constant.vi"() -> ("Module Name"=w711:string)  [unwired: 11 in]
      n265 = Format Into String(format string="An error occurred during initialization. %s is no longer running.", w711) -> (resulting string=w709:string)  [unwired: 2 in, 1 out]
      n266 = Merge Errors(w707, w705) -> (w706:errorcluster)
      n267 = call "Error Reported.vi"("Additional Information"=w709, "Error"=w706) -> ()  [unwired: 9 in, 1 out]
    }
  }
  n268 = Merge Errors(w26, w33) -> (w25:errorcluster)
  n269 = call "Close Module.vi"("error in (no error)"=w25, "Module Admin in"=w34) -> ("error out"=w28:errorcluster, "External Launch"=w23:bool, "Module Admin out"=w27:refnum<class "Delacor_lib_QMH_Module Admin.lvclass">)  [unwired: 7 in]
  n270 = Unregister For Events(event registration refnum=w32, error in=w28) -> (error out=w24:errorcluster)
  "error out" <- w24
  n271 = case "External Launch?" shown="True" w23 {
    tunnel: w24 -> [_ w717]
    tunnel: w21 -> [_ w716]
    tunnel: w13 -> [_ w714]
    frame False {
    }
    frame True {
      n272 = call-dynamic <vilib>:"Close.vi"("Panel In"=w716) -> ("Error Out"=w715:errorcluster)  [unwired: 10 in]
      n273 = call <vilib>:"Close.vi"("error in (no error)"=w715, "Controller in"=w714) -> ("error out"=w713:errorcluster)  [unwired: 9 in]
      n274 = case shown="Error" w717 {
        tunnel: w713 -> [_ _]
        frame No Error {
        }
        frame Error {
          n275 = invoke class="VI" method="FP.Open"("Activate"=TRUE ("Activate?")) -> ()  [unwired: 4 in, 5 out]
        }
      }
    }
  }
  n276 = local write "Module Admin"(w27) -> ()
